vi "svx_SC Line Property Dialog.vi"(0 "Refnum":refnum<vi>, 1 "State In":T2={"X Scale"={"Name"="Horizontal", "format string"="%#.2g", "Major Color"=16777238, "Minor Color"=16777216, "Scale Visible"=TRUE, " Label Visible"=TRUE, "Grid Style"=1, "Maximum"=1.0, "Minimum"=-1.0}, "Y Scale"={"Name"="Vertical", "format string"="%#.2g", "Major Color"=16777238, "Minor Color"=16777216, "Scale Visible"=TRUE, " Label Visible"=TRUE, "Grid Style"=1, "Maximum"=1.0, "Minimum"=-1.0}, "Plot"={"Point Style"=0, "Line Width"=0, "Line Style"=0, "Plot Color"=16860, "Point/fill"=16860}, "Arrow Color"=16860, "Autoscale"=TRUE, "Property Name"=[], "Container Bounds"={"Width"=550, "Height"=313}, "Background color"=16777226, "Annotation List"=[], "Cursor"={"Cursor Point Style"=13, "Cursor Style"=4, "Cursor Line Width"=1, "Cursor Line Style"=0, "Cursor Color"=16711680, "Cursor Name Visible"=TRUE, "Cursor Visible"=TRUE, "Cursor Position"={"X"=0.0, "Y"=0.0}, "Cursor Index"=0, "Lock Cursor Name"=FALSE, "Cursor reference"=0.0}, "size"=0, "Boundary Color"=9868950, "Maximum"=1.0, "Marker Point Style"=2, "Maker Visible"=TRUE, "Marker Color"=16860, "pair strings []"=[], "clearance boundary"=[{"boundary"={"x axis"=0.0, "y axis"=0.0}, "start point"=enum."center"}], "Custom pair name"=FALSE, "selector.visible"=TRUE, "Cursor Release"=refnum, "Children Tags"=[], "open?"=TRUE, "pair index"=[], "Legend Width"=200, " Parents Tags"="", "Label"="", "Legend Background"=16777226, "Legend Font"=16777222, "scale fit"=2, "user strings []"=[], "Item Width"=0, "out of state queue"=refnum, "property nodes"=refnum, "Kind"=enum."X-Scale", "Scale Range Change"=refnum} caption="State" {"pair index" min=0; "Y Scale"."Minimum" min=0.0; "Y Scale"."Maximum" min=0.0; "X Scale"."Minimum" min=0.0; "X Scale"."Maximum" min=0.0}, 2 "Clearance Only?":bool, 5 "SC Line in":refnum<vi>, 7 "cursor info":refnum<vi>, 9 "Tree":refnum<vi>, 11 "Data":T1, 12 "Action in":T6 caption="Action") -> (3 "State Out":T2={"X Scale"={"Name"="Horizontal", "format string"="%#.2g", "Major Color"=16777238, "Minor Color"=16777216, "Scale Visible"=TRUE, " Label Visible"=TRUE, "Grid Style"=1, "Maximum"=1.0, "Minimum"=-1.0}, "Y Scale"={"Name"="Vertical", "format string"="%#.2g", "Major Color"=16777238, "Minor Color"=16777216, "Scale Visible"=TRUE, " Label Visible"=TRUE, "Grid Style"=1, "Maximum"=1.0, "Minimum"=-1.0}, "Plot"={"Point Style"=0, "Line Width"=0, "Line Style"=0, "Plot Color"=16860, "Point/fill"=16860}, "Arrow Color"=16860, "Autoscale"=TRUE, "Property Name"=[], "Container Bounds"={"Width"=550, "Height"=313}, "Background color"=16777226, "Annotation List"=[], "Cursor"={"Cursor Point Style"=13, "Cursor Style"=4, "Cursor Line Width"=1, "Cursor Line Style"=0, "Cursor Color"=16711680, "Cursor Name Visible"=TRUE, "Cursor Visible"=TRUE, "Cursor Position"={"X"=0.0, "Y"=0.0}, "Cursor Index"=0, "Lock Cursor Name"=FALSE, "Cursor reference"=0.0}, "size"=0, "Boundary Color"=9868950, "Maximum"=1.0, "Marker Point Style"=2, "Maker Visible"=TRUE, "Marker Color"=16860, "pair strings []"=[], "clearance boundary"=[{"boundary"={"x axis"=0.0, "y axis"=0.0}, "start point"=enum."center"}], "Custom pair name"=FALSE, "selector.visible"=TRUE, "Cursor Release"=refnum, "Children Tags"=[], "open?"=TRUE, "pair index"=[], "Legend Width"=200, " Parents Tags"="", "Label"="", "Legend Background"=16777226, "Legend Font"=16777222, "scale fit"=2, "user strings []"=[], "Item Width"=0, "out of state queue"=refnum, "property nodes"=refnum, "Kind"=enum."X-Scale", "Scale Range Change"=refnum} caption="State" {"pair index" min=0; "Y Scale"."Minimum" min=0.0; "Y Scale"."Maximum" min=0.0; "X Scale"."Minimum" min=0.0; "X Scale"."Maximum" min=0.0}, 14 "Action out":T6 caption="Action")   [LabVIEW 2017, in "SVX SC Line.xctl"]
uses:
  <vilib>/addons/_XControls/Shaft Centerline/SVX SC Line.xctl
  <vilib>/_xctls/Action.ctl
  <vilib>/addons/_XControls/Shaft Centerline/subVIs/svx_SC Line State.ctl
  <vilib>/addons/_XControls/Shaft Centerline/subVIs/svx_SC Line Bounds.ctl
  <vilib>/addons/_XControls/Shaft Centerline/subVIs/svx_SC Line Annotation List.ctl
  <vilib>/addons/_XControls/Shaft Centerline/subVIs/svx_SC Line OutState Queue.ctl
  <vilib>/addons/_XControls/Shaft Centerline/subVIs/svx_SC Line Data.ctl
  <vilib>/addons/_XControls/Shaft Centerline/subVIs/svx_SC Line Core States.ctl
  <vilib>/_xctls/XControlSupport.lvlib
panel:
  in  "Update Scale?":bool
  in  "Help":bool
  in  "Cancel":bool
  in  "OK":bool
  in  "Main Tab":T7(tab)
  in  "Legend Font.Color":u32(colorbox)=16777222 caption="Legend font"
  in  "Legend Background.Color":u32(colorbox)=16777226 caption="Legend background"
  in  "Background.Color":u32(colorbox)=16777226 caption="Background"
  in  "Direction.Color":u32(colorbox)=6618880 caption="Direction"
  in  "Label.Visible":bool=TRUE
  in  "Label.Text":string="Shaft Centerline"
  in  "Caption.Visible":bool
  in  "Caption.Text":string="Shaft Centerline"
  in  "Enable State":T8(radio)
  in  "Format Selection":u16(ring) items=["Horizontal (X-Axis)", "Vertical (Y-Axis)"]
  in  "Hide trailing zeros":bool=TRUE
  in  "Digits":u8=2
  in  "Precision Type":u16(ring) items=["Digits of precision", "Significant digits"]
  in  "Type":i32(listbox)=2
  in  "Plot.Point Style":T9={"OK Button 17"=TRUE, "OK Button"=FALSE, "OK Button 2"=FALSE, "OK Button 3"=FALSE, "OK Button 4"=FALSE, "OK Button 5"=FALSE, "OK Button 6"=FALSE, "OK Button 7"=FALSE, "OK Button 8"=FALSE, "OK Button 9"=FALSE, "OK Button 10"=FALSE, "OK Button 11"=FALSE, "OK Button 12"=FALSE, "OK Button 13"=FALSE, "OK Button 14"=FALSE, "OK Button 15"=FALSE, "OK Button 16"=FALSE} caption="Point Style"
  in  "Line.Color":u32(colorbox) caption="Line"
  in  "Plot.Line Style":T10={"OK Button"=TRUE, "OK Button 2"=FALSE, "OK Button 3"=FALSE, "OK Button 4"=FALSE, "OK Button 5"=FALSE} caption="Line Style"
  in  "Plot.Line Width":T11={"OK Button 2"=TRUE, "OK Button 3"=FALSE, "OK Button 4"=FALSE, "OK Button 5"=FALSE, "OK Button 6"=FALSE, "OK Button 7"=FALSE} caption="Line Width"
  in  "Point/Fill.Color":u32(colorbox)=16777226 caption="Point/Fill"
  in  "Marker.Point Style":T9 caption="Cursor Point Style"
  in  "Marker Color":u32(colorbox) caption="Marker"
  in  "Marker.Visible":bool=TRUE caption="Show marker"
  in  "YGrid Style":u16(ring) caption="Grid Style and Colors"
  in  "XGrid Style":u16(ring) caption="Grid Style and Colors"
  in  "Minor Grid.Color":u32(colorbox)=13056 caption="Minor grid"
  in  "Major Grid.Color":u32(colorbox)=26112 caption="Major grid"
  in  "Scale Label.Visible":bool caption="Show scale label"
  in  "Maximum":dbl=10.0 format="%0.2f"
  in  "Minimum":dbl format="%0.2f"
  in  "Scale Fit":bool caption="Autoscale"
  in  "Scale.Visible":bool=TRUE caption="Show scale"
  in  "Scale Name":string caption="Name"
  in  "Scale Selection":u16(ring) items=["Horizontal (X-Axis)", "Vertical (Y-Axis)"]
  in  "Cursor Info Position.Lock":bool=TRUE
  in  "Cursor.Line Width":T11 caption="Cursor Line Width"
  in  "Cursor.Point Style":T9 caption="Cursor Point Style"
  in  "Cursor.Line Style":T10 caption="Cursor Line Style"
  in  "Cursor Info.Visible":bool caption="Show name"
  in  "Cursor.Style":T12 caption="Cursor Style"
  in  "Cursor.Color":u32(colorbox) caption="Cursor color"
  in  "Cursor.Visible":bool=TRUE
  in  "Pair Selection":u16(ring)
  in  "Start Point":u16(ring)=2 caption="Start point" items=["Center", "Top", "Bottom"]
  in  "X Axis":dbl=0.02 caption="X axis" min=0.0
  in  "Y Axis":dbl=0.02 caption="Y axis" min=0.0
  in  "Clearance Boundary.Color":u32(colorbox)=14847 caption="Clearance boundary"
  in  "Tip strip":string
  in  "Description":string
  # "Caption"
  # "Label"
  # "Enabled State"
  # "Color Scheme"
  # "Shaft Centerline"
  # "Colors"
  # "Marker"
  # "Cursor"
  # "Boundary"
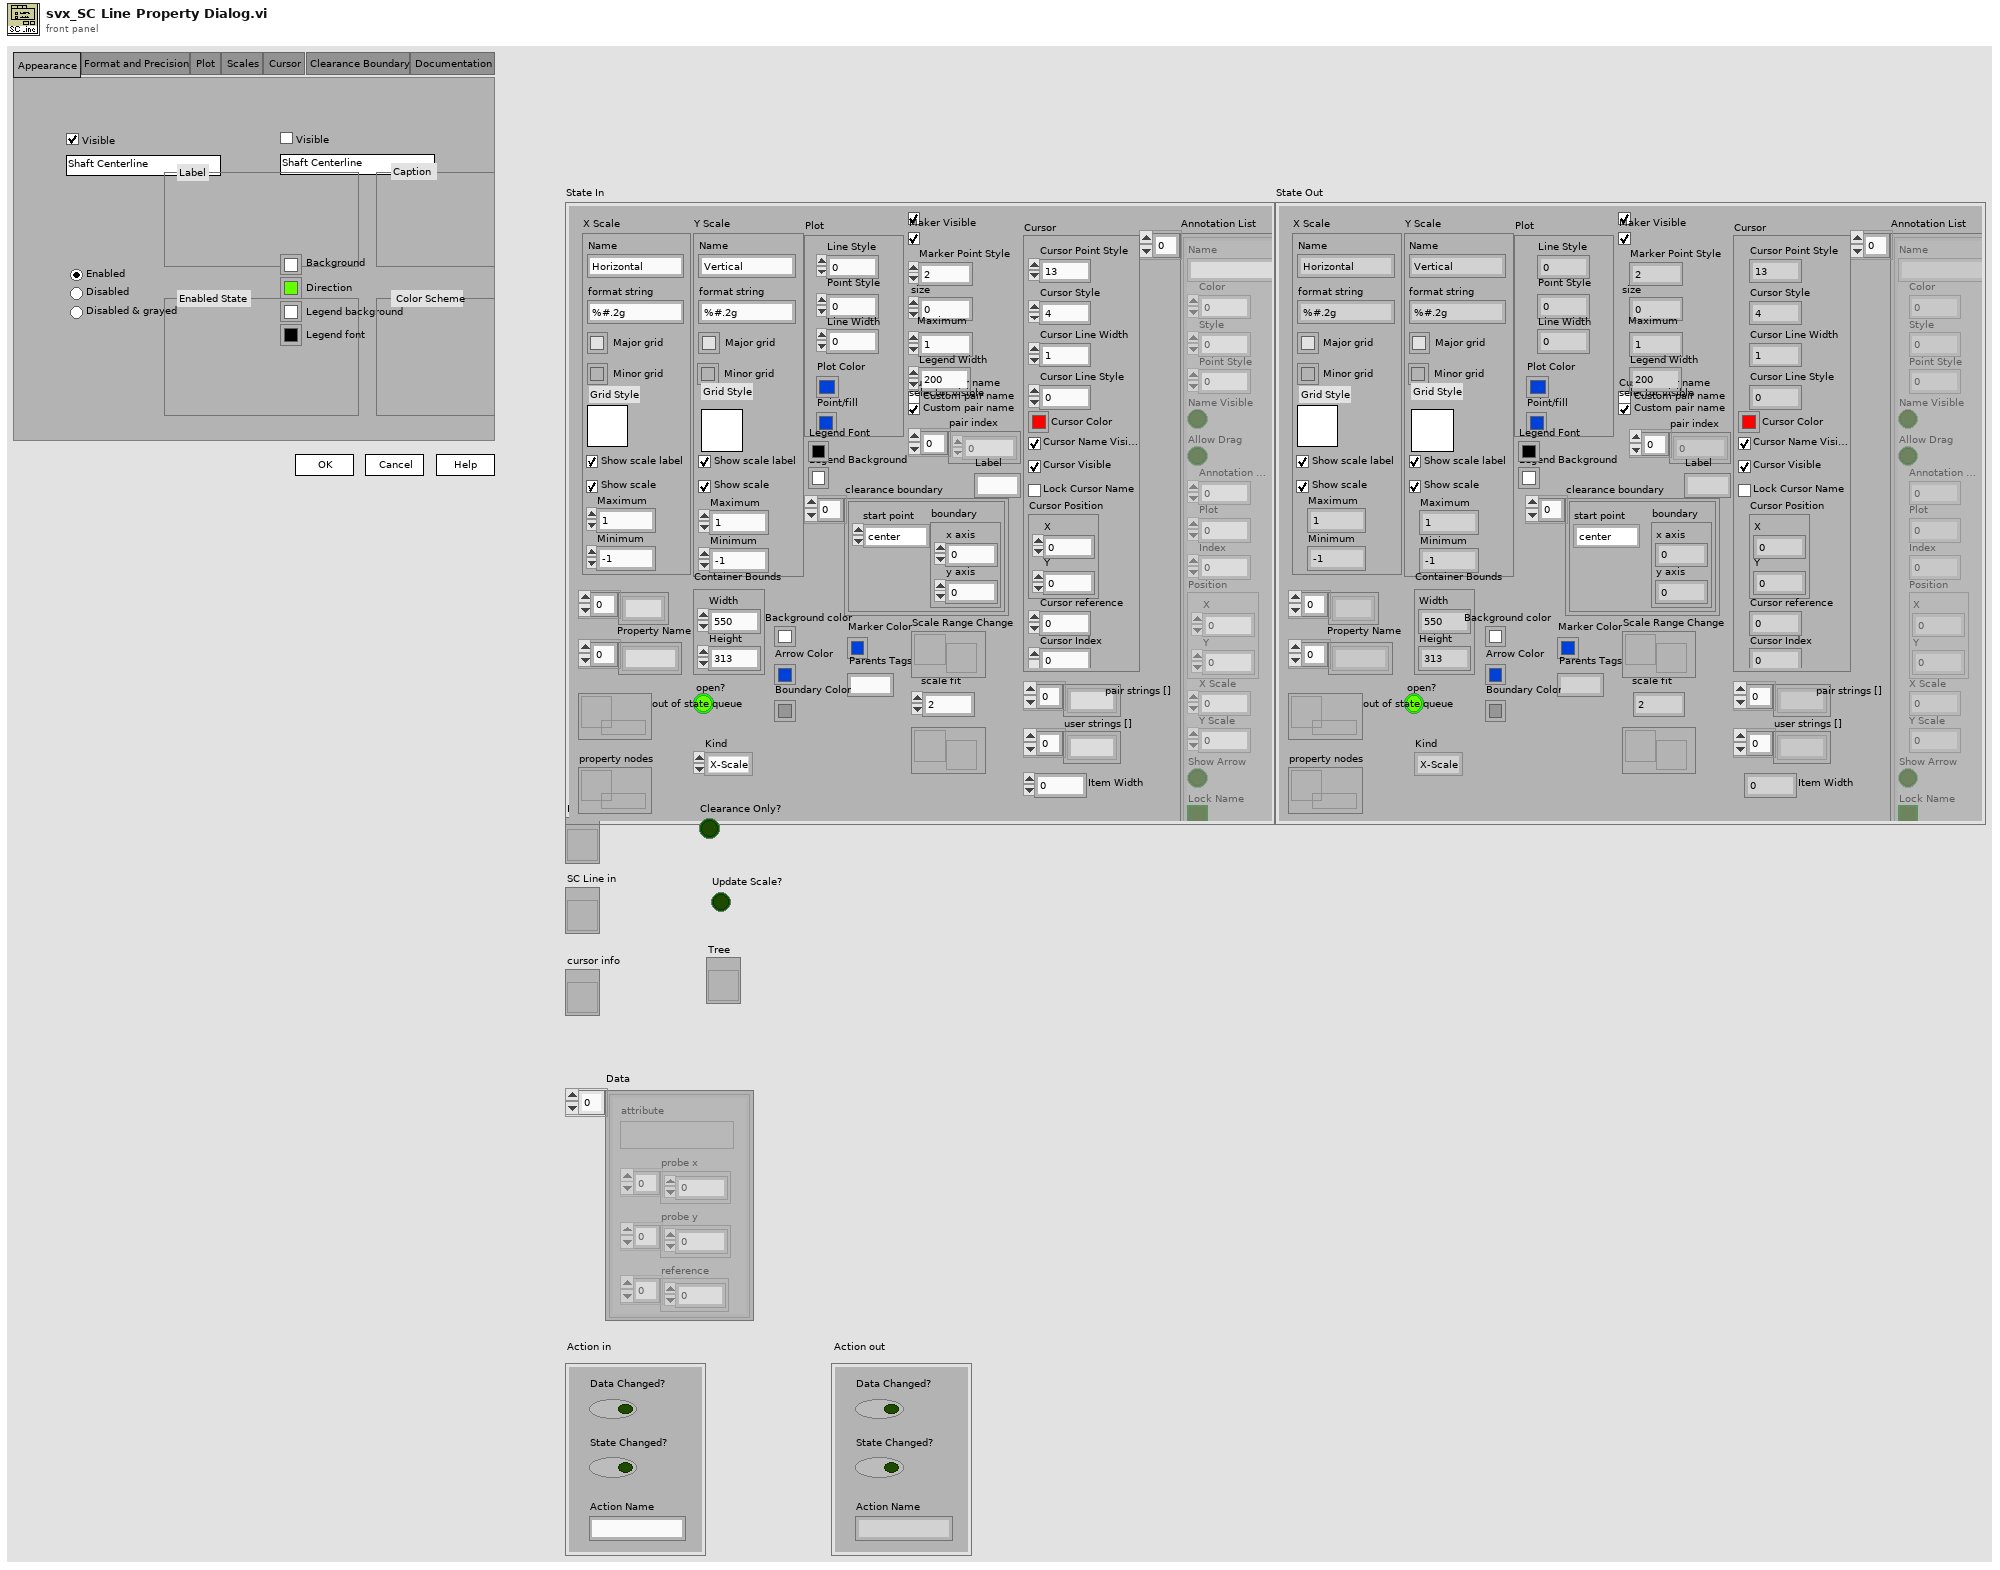
[diagram p1: front panel]
types:
  T1 = typedef "SVX SC Line.xctl/svx_SC Line Data.ctl" = cluster{"probe x":dbl[], "probe y":dbl[], "reference":dbl[], "attribute":variant}[]
  T2 = typedef "SVX SC Line.xctl/svx_SC Line State.ctl" = cluster{"X Scale":cluster{"Name":string, "format string":string, "Major Color":u32, "Minor Color":u32, "Scale Visible":bool, " Label Visible":bool, "Grid Style":u16, "Maximum":dbl, "Minimum":dbl}, "Y Scale":cluster{"Name":string, "format string":string, "Major Color":u32, "Minor Color":u32, "Scale Visible":bool, " Label Visible":bool, "Grid Style":u16, "Maximum":dbl, "Minimum":dbl}, "Plot":cluster{"Point Style":u8, "Line Width":u8, "Line Style":u8, "Plot Color":u32, "Point/fill":u32}, "Arrow Color":u32, "Autoscale":bool, "Property Name":string[], "Container Bounds":T3, "Background color":u32, "Annotation List":T4, "Cursor":cluster{"Cursor Point Style":u8, "Cursor Style":u8, "Cursor Line Width":u8, "Cursor Line Style":u8, "Cursor Color":u32, "Cursor Name Visible":bool, "Cursor Visible":bool, "Cursor Position":cluster{"X":dbl, "Y":dbl}, "Cursor Index":i32, "Lock Cursor Name":bool, "Cursor reference":dbl}, "size":i32, "Boundary Color":u32, "Maximum":dbl, "Marker Point Style":u8, "Maker Visible":bool, "Marker Color":u32, "pair strings []":string[], "clearance boundary":cluster{"boundary":cluster{"x axis":dbl, "y axis":dbl}, "start point":enum16{"center", "top", "bottom"}}[], "Custom pair name":bool, "selector.visible":bool, "Cursor Release":refnum<user-event>, "Children Tags":string[], "open?":bool, "pair index":i32[], "Legend Width":u32, " Parents Tags":string, "Label":string, "Legend Background":u32, "Legend Font":u32, "scale fit":u8, "user strings []":string[], "Item Width":u32, "out of state queue":T5, "property nodes":refnum<queue>, "Kind":enum16{"X-Scale", "Y-Scale", "Z-Scale"}, "Scale Range Change":refnum<user-event>}
  T3 = typedef "SVX SC Line.xctl/svx_SC Line Bounds.ctl" = cluster{"Width":u32, "Height":u32}
  T4 = typedef "SVX SC Line.xctl/svx_SC Line Annotation List.ctl" = cluster{"Name":string, "Color":u32, "Style":u8, "Point Style":u8, "Name Visible":bool, "Allow Drag":bool, "Annotation Mode":u32, "Plot":i32, "Index":i32, "Position":cluster{"X":dbl, "Y":dbl}, "X Scale":u32, "Y Scale":u32, "Show Arrow":bool, "Lock Name":bool, "Plot Area":i32, "Label Offset":cluster{"X":dbl, "Y":dbl}}[]
  T5 = typedef "SVX SC Line.xctl/svx_SC Line OutState Queue.ctl" = refnum<queue>
  T6 = typedef "XControlSupport.lvlib/Action.ctl" = cluster{"Data Changed?":bool, "State Changed?":bool, "Action Name":string}
  T7 = enum32{"Appearance", "Format and Precision", "Plot", "Scales", "Cursor", "Clearance Boundary", "Documentation"}
  T8 = enum32{"Enabled", "Disabled", "Disabled & grayed"}
  T9 = cluster{"OK Button 17":bool, "OK Button":bool, "OK Button 2":bool, "OK Button 3":bool, "OK Button 4":bool, "OK Button 5":bool, "OK Button 6":bool, "OK Button 7":bool, "OK Button 8":bool, "OK Button 9":bool, "OK Button 10":bool, "OK Button 11":bool, "OK Button 12":bool, "OK Button 13":bool, "OK Button 14":bool, "OK Button 15":bool, "OK Button 16":bool}
  T10 = cluster{"OK Button":bool, "OK Button 2":bool, "OK Button 3":bool, "OK Button 4":bool, "OK Button 5":bool}
  T11 = cluster{"OK Button 2":bool, "OK Button 3":bool, "OK Button 4":bool, "OK Button 5":bool, "OK Button 6":bool, "OK Button 7":bool}
  T12 = cluster{"OK Button 17":bool, "OK Button":bool, "OK Button 2":bool, "OK Button 5":bool, "OK Button 13":bool, "OK Button 10":bool, "OK Button 6":bool, "OK Button 9":bool, "OK Button 14":bool}
  T13 = cluster{"boundary":cluster{"x axis":dbl, "y axis":dbl}, "start point":enum16{"center", "top", "bottom"}}[]
  T14 = cluster{"boundary":cluster{"x axis":dbl, "y axis":dbl}, "start point":enum16{"center", "top", "bottom"}}
  T15 = cluster{"Desc":string, "TipStrip":string, "Label.Text":string, "Label.Visible":bool, "Caption.Text":string, "Caption.Visible":bool, "Disabled":u8}
  T16 = cluster{"Refnum":refnum<vi>, "SC Line in":refnum<vi>, "cursor info":refnum<vi>, "Tree":refnum<vi>, "This VI":refnum<vi>}
  T17 = typedef "SVX SC Line.xctl/svx_SC Line Core States.ctl" = enum16{"None", "[Axis] Autoscale", "[Image] Update", "[Cursor] Name", "[Plot] Grid&BG", "[Marker] Update", "[Tree] Tags", "[Data] Update", "[Layout] Size", "[Tree] Checkbox", "[Tree] Visible", "[Tree] Open", "[Axis] X", "[Axis] Y", "[Plot] Color", "[Axis] Format String", "[Data] Compare Strings", "[Cursor] Apearance", "[Axis] Name&Visible", "[Tree] Color", "[Data] Index", "[Cursor] Index", "[Axis] Event"}
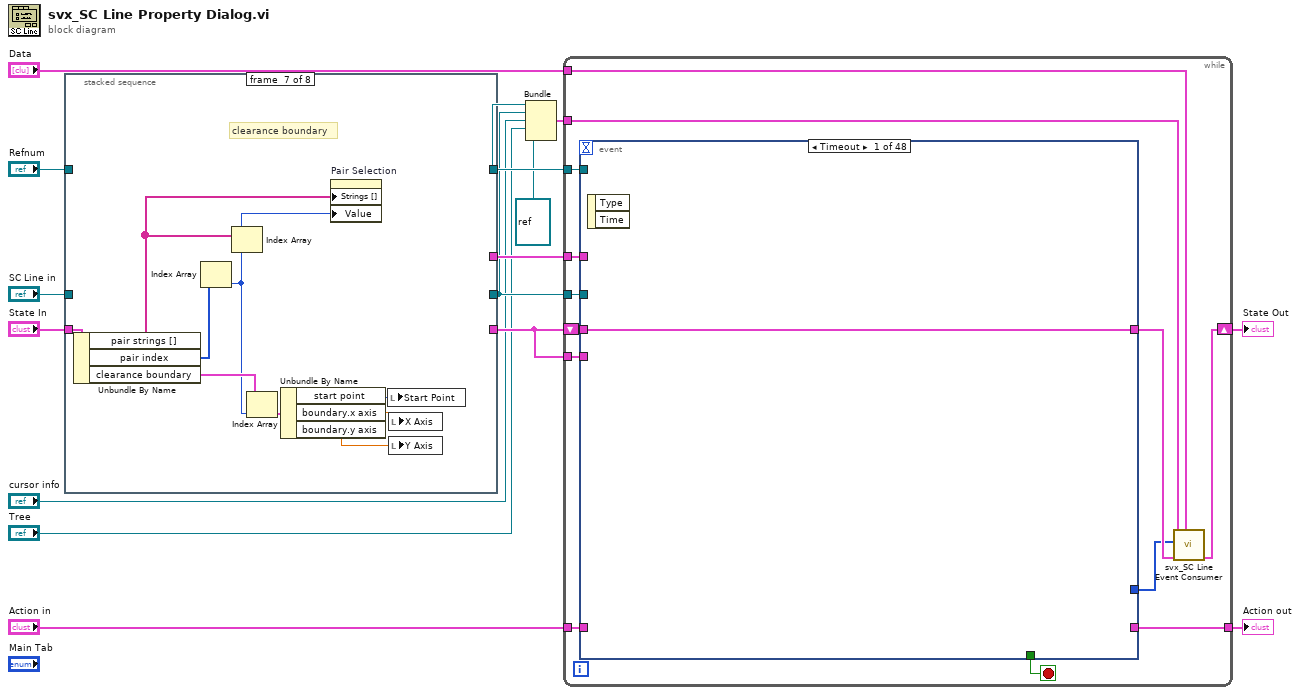
[diagram p0: block diagram]
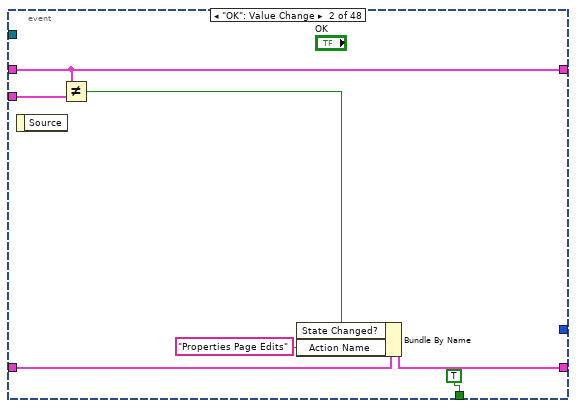
[diagram p2: hidden frame]
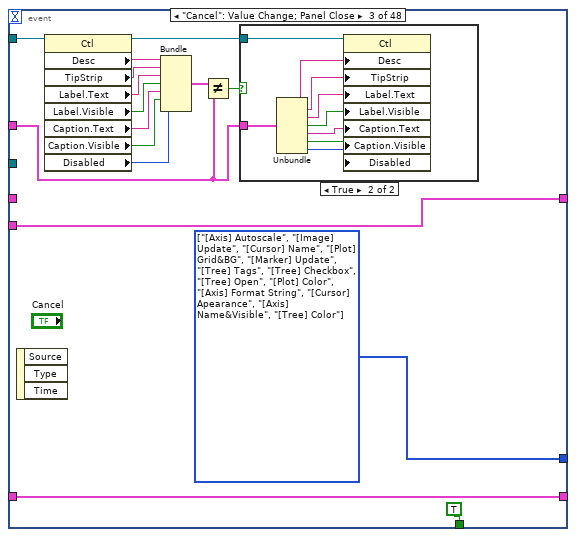
[diagram p3: hidden frame]
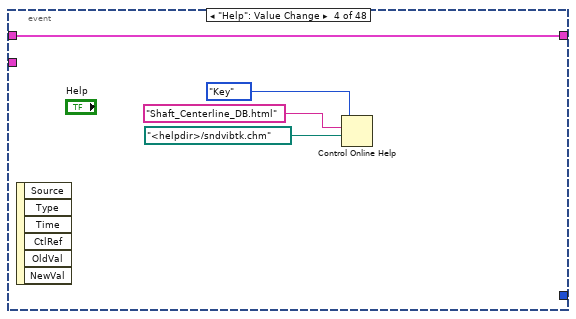
[diagram p5: hidden frame]
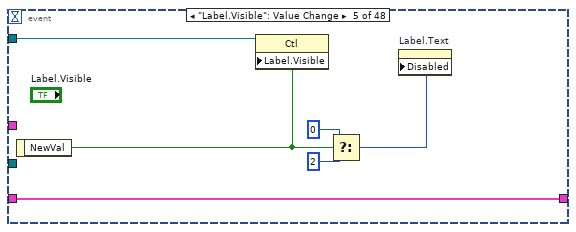
[diagram p6: hidden frame]
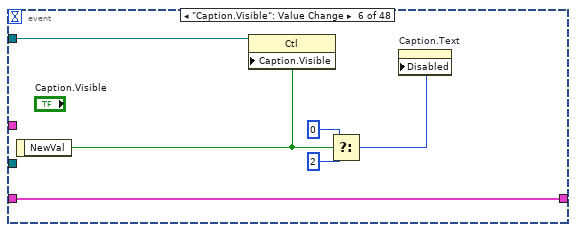
[diagram p7: hidden frame]
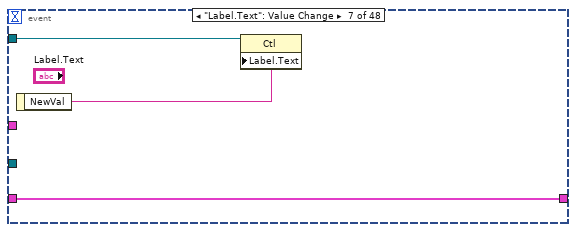
[diagram p8: hidden frame]
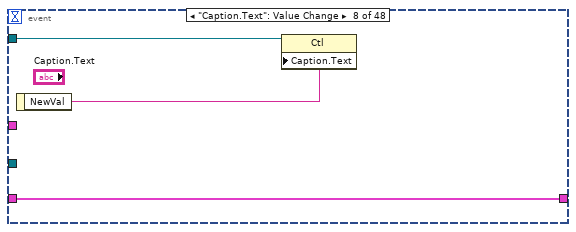
[diagram p9: hidden frame]
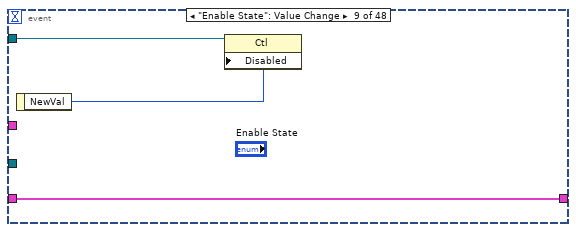
[diagram p10: hidden frame]
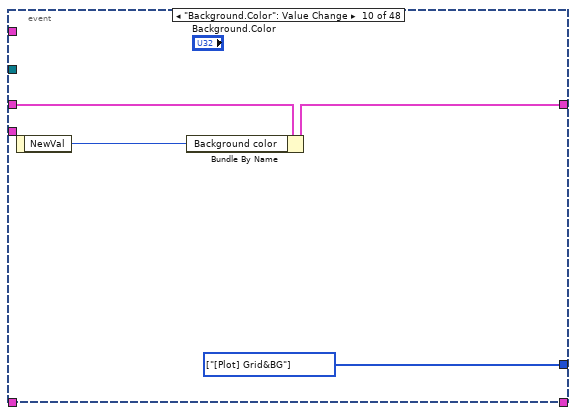
[diagram p11: hidden frame]
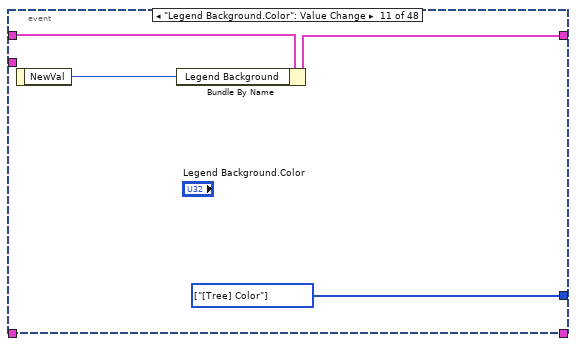
[diagram p12: hidden frame]
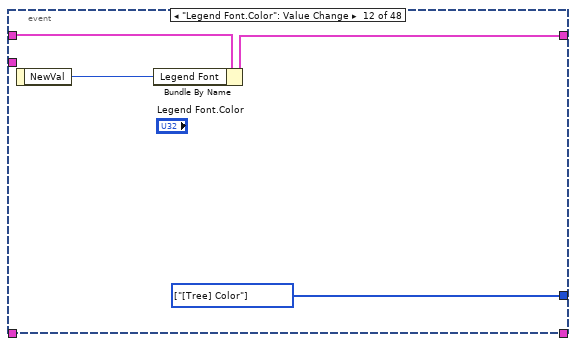
[diagram p13: hidden frame]
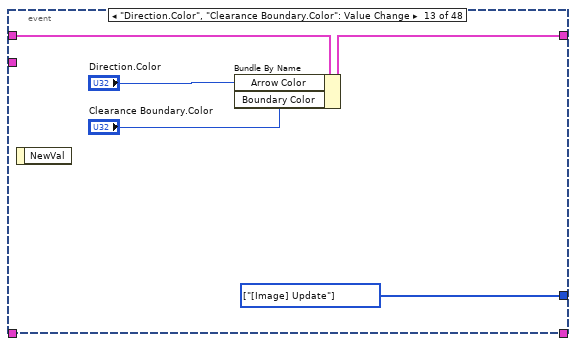
[diagram p14: hidden frame]
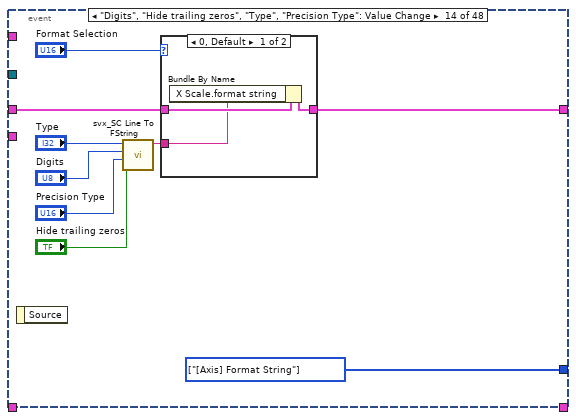
[diagram p15: hidden frame]
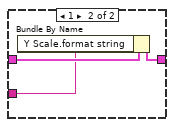
[diagram p16: hidden frame]
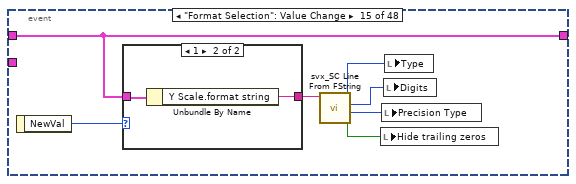
[diagram p17: hidden frame]
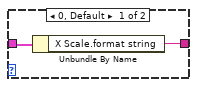
[diagram p18: hidden frame]
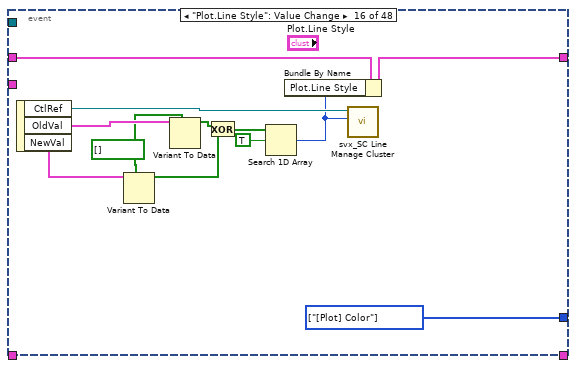
[diagram p19: hidden frame]
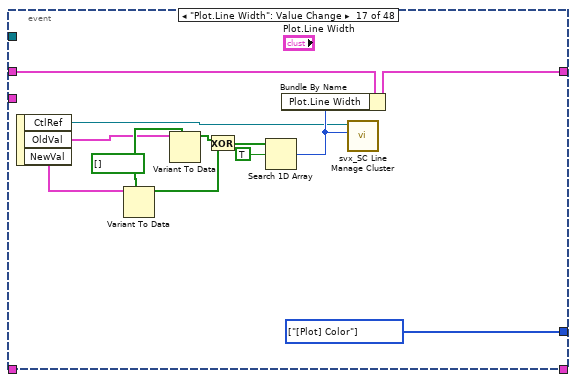
[diagram p20: hidden frame]
diagram:
  n1 = stacked-sequence {
    tunnel: "Refnum" -> [_ w47 _ _ _ _ _ w144]
    tunnel: [_ _ _ _ _ _ _ w143] -> w6
    tunnel: [_ _ _ _ _ _ _ w140] -> w14
    tunnel: [_ _ _ _ _ _ _ w141] -> w5
    tunnel: "SC Line in" -> [_ _ _ _ _ _ _ w141]
    tunnel: [_ _ _ _ _ _ _ w142] -> w11
    tunnel: "State In" -> [_ w30 w48 w58 w67 w100 w124 w140]
    frame #0 {
      n2 = property on="Main Tab" class="TabCtl (strict)"() -> ("Pages"=w18:refnum<vi>[])  [unwired: 2 in, 2 out]
      n3 = case shown="True" "Clearance Only?" {
        tunnel: w18 -> [w21 w27]
        tunnel: [T7."Clearance Boundary" ("Main Tab") T7."Appearance" ("Main Tab")] -> w17
        frame True {
          n4 = for {
            tunnel: w21 -> [w25] mode=indexing
            i -> [w24]
            n5 = Equal?(x=5, y=w24) -> (x = y?=w22:bool)
            n6 = property on="Property Node" class="Page"(reference=w25, "PageVis"=w22) -> ()  [unwired: 1 in, 2 out]
          }
        }
        frame False {
          n7 = for {
            tunnel: w27 -> [w29] mode=indexing
            n8 = property on="Property Node" class="Page"(reference=w29, "PageVis"=TRUE ("Page Visible")) -> ()  [unwired: 1 in, 2 out]
          }
        }
      }
      n9 = local write "Main Tab"(w17) -> ()
      n10 = local write "Update Scale?"(FALSE ("Update Scale?")) -> ()
    }
    frame #1 {
      # "Appearance"
      n11 = Unbundle By Name(w30) -> ("Background color"=w46:u32, "Arrow Color"=w45:u32, "Boundary Color"=w33:u32, "Legend Background"=w32:u32, "Legend Font"=w31:u32)
      n12 = property class="Ctl"(reference=w47) -> ("Label.Text"=w39:string, "Label.Visible"=w38:bool, "Caption.Text"=w37:string, "Caption.Visible"=w35:bool, "Disabled"=w36:u8)  [unwired: 1 in, 2 out]
      n13 = local write "Clearance Boundary.Color"(w33) -> ()
      n14 = local write "Background.Color"(w46) -> ()
      n15 = local write "Legend Font.Color"(w31) -> ()
      n16 = local write "Caption.Text"(w37) -> ()
      n17 = local write "Label.Text"(w39) -> ()
      n18 = local write "Enable State"(w36) -> ()
      n19 = local write "Caption.Visible"(w35) -> ()
      n20 = local write "Label.Visible"(w38) -> ()
      n21 = local write "Legend Background.Color"(w32) -> ()
      n22 = local write "Direction.Color"(w45) -> ()
      n23 = Select(t=u8 0 ("Disabled"), s=w38, f=u8 2) -> (s? t:f=w43:u8)
      n24 = Select(t=u8 0 ("Disabled"), s=w35, f=u8 2) -> (s? t:f=w40:u8)
      n25 = property on="Label.Text" class="Str"("Disabled"=w43) -> ()  [unwired: 2 in, 2 out]
      n26 = property on="Caption.Text" class="Str"("Disabled"=w40) -> ()  [unwired: 2 in, 2 out]
    }
    frame #2 {
      w54 = u16 0 items=["X-Axis", "Y-Axis"] ("Format selection")
      # "Format and Precision"
      n27 = Unbundle By Name(w48) -> ("X Scale.format string"=w53:string)
      n28 = call <vilib>:"svx_SC Line From FString.vi"("Format string"=w53) -> ("trailing zeros"=w49:bool, "Precision Type"=w50:u16, "Digits"=w51:u8, "Type"=w52:i32)  [unwired: 7 in]
      n29 = local write "Format Selection"(w54) -> ()
      n30 = local write "Hide trailing zeros"(w49) -> ()
      n31 = local write "Precision Type"(w50) -> ()
      n32 = local write "Digits"(w51) -> ()
      n33 = local write "Type"(w52) -> ()
    }
    frame #3 {
      # "Plot"
      n34 = Unbundle By Name(w58) -> ("Plot.Plot Color"=w60:u32, "Plot.Point/fill"=w59:u32, "Plot.Line Width"=w66:u8, "Plot.Line Style"=w64:u8, "Plot.Point Style"=w63:u8)
      n35 = control-ref of="Plot.Line Width"() -> (w65:refnum<vi>)
      n36 = control-ref of="Plot.Line Style"() -> (w61:refnum<vi>)
      n37 = control-ref of="Plot.Point Style"() -> (w62:refnum<vi>)
      n38 = local write "Line.Color"(w60) -> ()
      n39 = To Long Integer(number=w66) -> (32bit integer=w55:i32)
      n40 = To Long Integer(number=w64) -> (32bit integer=w56:i32)
      n41 = To Long Integer(number=w63) -> (32bit integer=w57:i32)
      n42 = local write "Point/Fill.Color"(w59) -> ()
      n43 = call <vilib>:"svx_SC Line Manage Cluster.vi"("index"=w55, "Clust Refnum"=w65) -> ()  [unwired: 10 in]
      n44 = call <vilib>:"svx_SC Line Manage Cluster.vi"("index"=w56, "Clust Refnum"=w61) -> ()  [unwired: 10 in]
      n45 = call <vilib>:"svx_SC Line Manage Cluster.vi"("index"=w57, "Clust Refnum"=w62) -> ()  [unwired: 10 in]
    }
    frame #4 {
      w90 = u16 0 items=["X-Axis", "Y-Axis"] ("Scale selection")
      # "Scales"
      n46 = Unbundle By Name(w67) -> ("Y Scale.Name"=w73:string, "X Scale.Name"=w71:string, "X Scale.Label Visible"=w89:bool, "X Scale.Scale Visible"=w88:bool, "X Scale.Grid Style"=w78:u16, "X Scale.Major Color"=w87:u32, "X Scale.Minor Color"=w86:u32, "Autoscale"=w83:bool, "X Scale.Minimum"=w76:dbl, "X Scale.Maximum"=w75:dbl)
      n47 = property on="YGrid Style" class="Ring (strict)"("Visible"=FALSE) -> ()  [unwired: 2 in, 2 out]
      n48 = property on="XGrid Style" class="Ring (strict)"("Visible"=TRUE) -> ()  [unwired: 2 in, 2 out]
      n49 = Concatenate Strings(w73, " (Y-Axis)" ("string")) -> (w69:string)
      n50 = Concatenate Strings(w71, " (X-Axis)" ("string")) -> (w70:string)
      n51 = local write "Minimum"(w76) -> ()
      n52 = local write "Scale Label.Visible"(w89) -> ()
      n53 = local write "Maximum"(w75) -> ()
      n54 = local write "Minor Grid.Color"(w86) -> ()
      n55 = local write "XGrid Style"(w78) -> ()
      n56 = local write "Scale Selection"(w90) -> ()
      n57 = case shown="0, Default" w78 {
        tunnel: [w91 u8 0 ("Disabled") w94] -> w80
        tunnel: [w91 u8 2 ("Disabled") w94] -> w79
        frame 0, Default {
          w91 = u8 2 ("Disabled")
        }
        frame 1 {
        }
        frame 2 {
          w94 = u8 0 ("Disabled")
        }
      }
      n58 = Build Array(w70, w69) -> (w68:string[])
      n59 = property on="Scale Selection" class="Ring (strict)"("Strings []"=w68) -> ()  [unwired: 2 in, 2 out]
      n60 = property on="Format Selection" class="Ring (strict)"("Strings []"=w68) -> ()  [unwired: 2 in, 2 out]
      n61 = Select(t=u8 2 ("Disabled"), s=w83, f=u8 0) -> (s? t:f=w82:u8)
      n62 = local write "Scale Name"(w71) -> ()
      n63 = local write "Scale.Visible"(w88) -> ()
      n64 = local write "Major Grid.Color"(w87) -> ()
      n65 = local write "Scale Fit"(w83) -> ()
      n66 = property on="Minimum" class="DigNum (strict)"("Disabled"=w82) -> ()  [unwired: 2 in, 2 out]
      n67 = property on="Maximum" class="DigNum (strict)"("Disabled"=w82) -> ()  [unwired: 2 in, 2 out]
      n68 = property on="Major Grid.Color" class="ColBox"("Disabled"=w80) -> ()  [unwired: 2 in, 2 out]
      n69 = property on="Minor Grid.Color" class="ColBox"("Disabled"=w79) -> ()  [unwired: 2 in, 2 out]
    }
    frame #5 {
      # "Cursor"
      n70 = Unbundle By Name(w100) -> ("Cursor.Cursor Point Style"=w123:u8, "Cursor.Cursor Style"=w121:u8, "Cursor.Cursor Line Width"=w119:u8, "Cursor.Cursor Line Style"=w117:u8, "Cursor.Cursor Color"=w115:u32, "Cursor.Cursor Name Visible"=w102:bool, "Cursor.Cursor Visible"=w103:bool, "Marker Point Style"=w114:u8, "Maker Visible"=w112:bool, "Marker Color"=w111:u32, "Cursor.Lock Cursor Name"=w110:bool)
      n71 = And(x=w103, y=w102) -> (x .and. y?=w101:bool)
      n72 = Select(t=u8 0 ("Disabled"), s=w101, f=u8 2) -> (s? t:f=w104:u8)
      n73 = Select(t=u8 0 ("Disabled"), s=w103, f=u8 2) -> (s? t:f=w107:u8)
      n74 = property on="Cursor Info.Visible" class="Bool (strict)"("Disabled"=w107) -> ()  [unwired: 2 in, 2 out]
      n75 = property on="Cursor Info Position.Lock" class="Bool (strict)"("Disabled"=w104) -> ()  [unwired: 2 in, 2 out]
      n76 = local write "Cursor Info Position.Lock"(w110) -> ()
      n77 = local write "Cursor.Visible"(w103) -> ()
      n78 = local write "Marker.Visible"(w112) -> ()
      n79 = local write "Cursor.Color"(w115) -> ()
      n80 = To Long Integer(number=w121) -> (32bit integer=w96:i32)
      n81 = To Long Integer(number=w117) -> (32bit integer=w98:i32)
      n82 = control-ref of="Cursor.Point Style"() -> (w122:refnum<vi>)
      n83 = control-ref of="Cursor.Style"() -> (w120:refnum<vi>)
      n84 = control-ref of="Cursor.Line Style"() -> (w116:refnum<vi>)
      n85 = call <vilib>:"svx_SC Line Manage Cluster.vi"("index"=w96, "Clust Refnum"=w120) -> ()  [unwired: 10 in]
      n86 = call <vilib>:"svx_SC Line Manage Cluster.vi"("index"=w98, "Clust Refnum"=w116) -> ()  [unwired: 10 in]
      n87 = To Long Integer(number=w119) -> (32bit integer=w97:i32)
      n88 = To Long Integer(number=w114) -> (32bit integer=w99:i32)
      n89 = local write "Cursor Info.Visible"(w102) -> ()
      n90 = To Long Integer(number=w123) -> (32bit integer=w95:i32)
      n91 = control-ref of="Marker.Point Style"() -> (w113:refnum<vi>)
      n92 = local write "Marker Color"(w111) -> ()
      n93 = control-ref of="Cursor.Line Width"() -> (w118:refnum<vi>)
      n94 = call <vilib>:"svx_SC Line Manage Cluster.vi"("index"=w99, "Clust Refnum"=w113) -> ()  [unwired: 10 in]
      n95 = call <vilib>:"svx_SC Line Manage Cluster.vi"("index"=w95, "Clust Refnum"=w122) -> ()  [unwired: 10 in]
      n96 = call <vilib>:"svx_SC Line Manage Cluster.vi"("index"=w97, "Clust Refnum"=w118) -> ()  [unwired: 10 in]
    }
    frame #6 {
      # "clearance boundary"
      n97 = Unbundle By Name(w124) -> ("pair strings []"=w125:string[], "pair index"=w127:i32[], "clearance boundary"=w132:T13)
      n98 = Index Array(array=w127) -> (element=w126:i32)  [unwired: 1 in]
      n99 = Index Array(array=w125, index=w126) -> ()  [unwired: 1 out]
      n100 = Index Array(array=w132, index=w126) -> (element=w131:T14)
      n101 = Unbundle By Name(w131) -> ("start point"=w130:enum16{"center", "top", "bottom"}, "boundary.x axis"=w128:dbl, "boundary.y axis"=w129:dbl)
      n102 = property on="Pair Selection" class="Ring (strict)"("Strings []"=w125, "Value"=w126) -> ()  [unwired: 2 in, 2 out]
      n103 = local write "Start Point"(w130) -> ()
      n104 = local write "X Axis"(w128) -> ()
      n105 = local write "Y Axis"(w129) -> ()
    }
    frame #7 {
      n106 = property class="Ctl"(reference=w144) -> (reference out=w143:refnum<vi>, "Desc"=w133:string, "TipStrip"=w134:string, "Label.Text"=w139:string, "Label.Visible"=w138:bool, "Caption.Text"=w137:string, "Caption.Visible"=w136:bool, "Disabled"=w135:u8)  [unwired: 1 in, 1 out]
      n107 = local write "Description"(w133) -> ()
      n108 = local write "Tip strip"(w134) -> ()
      n109 = Bundle("Desc"=w133, "TipStrip"=w134, "Label.Text"=w139, "Label.Visible"=w138, "Caption.Text"=w137, "Caption.Visible"=w136, "Disabled"=w135) -> (w142:T15)  [unwired: 1 in]
    }
  }
  n110 = Bundle("Refnum"=w6, "SC Line in"=w5, "cursor info"="cursor info", "Tree"="Tree", "This VI"=refnum<vi> refnum) -> (w4:T16)  [unwired: 1 in]
  n111 = while {
    tunnel: w6 -> [w147]
    shift-right: [w150] -> w10
    shift-left: w14 -> [w156]
    tunnel: w14 -> [w153]
    tunnel: "Action in" -> [w152]
    tunnel: [w155] -> w12
    tunnel: w5 -> [w146]
    tunnel: w11 -> [w154]
    tunnel: "Data" -> [w148]
    tunnel: w4 -> [w145]
    stop <- w157 stop-if-true
    n112 = event shown="[0] Timeout" {
      selector: _ -> [_ _ _ _ _ _ _ _ _ _ _ _ _ _ _ _ _ _ _ _ _ _ _ _ _ _ _ _ _ _ _ _ _ _ _ _ _ _ _ _ _ _ _ _ _ _ _ _]
      dyn-events: _ -> [_ _ _ _ _ _ _ _ _ _ _ _ _ _ _ _ _ _ _ _ _ _ _ _ _ _ _ _ _ _ _ _ _ _ _ _ _ _ _ _ _ _ _ _ _ _ _ _]
      timeout: _ -> [_ _ _ _ _ _ _ _ _ _ _ _ _ _ _ _ _ _ _ _ _ _ _ _ _ _ _ _ _ _ _ _ _ _ _ _ _ _ _ _ _ _ _ _ _ _ _ _]
      tunnel: [_ TRUE TRUE _ _ _ _ _ _ _ _ _ _ _ _ _ _ _ _ _ _ _ _ _ _ _ _ _ _ _ _ _ _ _ _ _ _ _ _ _ _ _ _ _ _ _ _ _] -> w157
      tunnel: w156 -> [w158 w159 _ w191 w195 w201 w207 w210 w213 w219 w223 w227 w229 w235 w253 w262 w277 w289 w298 w302 w311 w324 w335 w351 w366 w386 w396 w406 w417 w427 w474 w486 w498 w510 w522 w526 w538 w542 w549 w558 w562 w573 w588 w603 w608 w615 w618 w621]
      tunnel: w153 -> [_ w164 w179 _ _ _ _ _ _ _ _ _ _ _ _ _ _ _ _ _ _ _ _ _ _ _ _ _ _ _ _ _ _ _ _ _ _ _ _ _ _ _ _ _ _ _ _ _]
      tunnel: [_ w162 w181 _ _ _ _ _ _ _ _ _ _ _ _ _ _ _ _ _ _ _ _ _ _ _ _ _ _ _ _ _ _ _ _ _ _ _ _ _ _ _ _ _ _ _ _ _] -> w155
      tunnel: [_ _ w166 _ _ _ _ _ _ w216 w220 w224 w228 w233 _ w259 w271 w283 w295 w299 w303 w320 w331 w348 w364 w382 w392 w402 w413 _ w468 w480 w492 w504 w516 w523 w527 w539 w543 w555 w559 w568 w583 w598 _ _ _ _] -> w149
      tunnel: w146 -> [_ _ _ _ _ _ _ _ _ _ _ _ _ _ _ _ _ _ _ _ _ _ _ w349 _ _ _ _ _ _ _ _ _ _ _ _ _ _ _ _ _ _ _ _ _ _ _ _]
      tunnel: w147 -> [_ _ w178 _ w200 w206 w209 w212 w215 _ _ _ _ _ _ _ _ _ _ _ _ _ _ _ _ _ _ _ _ _ _ _ _ _ _ _ _ _ _ _ _ _ _ _ _ w617 w620 _]
      tunnel: w154 -> [_ _ w169 _ _ _ _ _ _ _ _ _ _ _ _ _ _ _ _ _ _ _ _ _ _ _ _ _ _ _ _ _ _ _ _ _ _ _ _ _ _ _ _ _ _ _ _ _]
      tunnel: [w158 w159 w179 w191 w195 w201 w207 w210 w213 w218 w222 w226 w232 w234 w253 w261 w276 w288 w297 w301 w310 w323 w334 w347 w365 w387 w397 w405 w416 w427 w473 w485 w497 w509 w521 w525 w537 w541 w548 w557 w561 w572 w587 w602 w608 w615 w618 w621] -> w151
      tunnel: w152 -> [_ w163 w181 _ _ _ _ _ _ _ _ _ _ _ _ _ _ _ _ _ _ _ _ _ _ _ _ _ _ _ _ _ _ _ _ _ _ _ _ _ _ _ _ _ _ _ _ _]
      event Timeout {
        n113 = event-data() -> ()  [unwired: 1 in, 2 out]
      }
      event "OK": Value Change {
        n114 = event-data() -> ()  [unwired: 1 in, 1 out]
        n115 = Not Equal?(x=w159, y=w164) -> (x != y?=w161:bool)
        n116 = Bundle By Name(cluster=w163, "State Changed?"=w161, "Action Name"="Properties Page Edits") -> (w162:T6)
      }
      event "Cancel": Value Change; Panel Close {
        w166 = T17[] [enum."[Axis] Autoscale", enum."[Image] Update", enum."[Cursor] Name", enum."[Plot] Grid&BG", enum."[Marker] Update", enum."[Tree] Tags", enum."[Tree] Checkbox", enum."[Tree] Open", enum."[Plot] Color", enum."[Axis] Format String", enum."[Cursor] Apearance", enum."[Axis] Name&Visible", enum."[Tree] Color"] items=["None", "[Axis] Autoscale", "[Image] Update", "[Cursor] Name", "[Plot] Grid&BG", "[Marker] Update", "[Tree] Tags", "[Data] Update", "[Layout] Size", "[Tree] Checkbox", "[Tree] Visible", "[Tree] Open", "[Axis] X", "[Axis] Y", "[Plot] Color", "[Axis] Format String", "[Data] Compare Strings", "[Cursor] Apearance", "[Axis] Name&Visible", "[Tree] Color", "[Data] Index", "[Cursor] Index", "[Axis] Event"]
        n117 = event-data() -> ()  [unwired: 1 in, 3 out]
        n118 = property class="Ctl"(reference=w178) -> (reference out=w168:refnum<vi>, "Desc"=w177:string, "TipStrip"=w176:string, "Label.Text"=w175:string, "Label.Visible"=w174:bool, "Caption.Text"=w173:string, "Caption.Visible"=w172:bool, "Disabled"=w171:u8)  [unwired: 1 in, 1 out]
        n119 = Bundle("Desc"=w177, "TipStrip"=w176, "Label.Text"=w175, "Label.Visible"=w174, "Caption.Text"=w173, "Caption.Visible"=w172, "Disabled"=w171) -> (w170:T15)  [unwired: 1 in]
        n120 = Not Equal?(x=w170, y=w169) -> (x != y?=w167:bool)
        n121 = case shown="True" w167 {
          tunnel: w169 -> [_ w190]
          tunnel: w168 -> [_ w182]
          frame False {
          }
          frame True {
            n122 = Unbundle(w190) -> ("Desc"=w189:string, "TipStrip"=w188:string, "Label.Text"=w187:string, "Label.Visible"=w186:bool, "Caption.Text"=w185:string, "Caption.Visible"=w184:bool, "Disabled"=w183:u8)
            n123 = property class="Ctl"(reference=w182, "Desc"=w189, "TipStrip"=w188, "Label.Text"=w187, "Label.Visible"=w186, "Caption.Text"=w185, "Caption.Visible"=w184, "Disabled"=w183) -> ()  [unwired: 1 in, 2 out]
          }
        }
      }
      event "Help": Value Change {
        n124 = event-data() -> ()  [unwired: 1 in, 6 out]
        n125 = Control Online Help(2:path "<helpdir>/sndvibtk.chm" ("Path to the help file"), 3:"Shaft_Centerline_DB.html" ("String to search for"), 4:enum16{"Contents", "Key", "Close"}."Key" ("Operation")) -> ()  [unwired: 1 in, 1 out]
      }
      event "Label.Visible": Value Change {
        n126 = event-data() -> ("NewVal"=w197:bool)  [unwired: 1 in]
        n127 = property class="Ctl"(reference=w200, "Label.Visible"=w197) -> ()  [unwired: 1 in, 2 out]
        n128 = Select(t=u8 0 ("Disabled"), s=w197, f=u8 2) -> (s? t:f=w196:u8)
        n129 = property on="Label.Text" class="Str"("Disabled"=w196) -> ()  [unwired: 2 in, 2 out]
      }
      event "Caption.Visible": Value Change {
        n130 = event-data() -> ("NewVal"=w203:bool)  [unwired: 1 in]
        n131 = property class="Ctl"(reference=w206, "Caption.Visible"=w203) -> ()  [unwired: 1 in, 2 out]
        n132 = Select(t=u8 0 ("Disabled"), s=w203, f=u8 2) -> (s? t:f=w202:u8)
        n133 = property on="Caption.Text" class="Str"("Disabled"=w202) -> ()  [unwired: 2 in, 2 out]
      }
      event "Label.Text": Value Change {
        n134 = event-data() -> ("NewVal"=w208:string)  [unwired: 1 in]
        n135 = property class="Ctl"(reference=w209, "Label.Text"=w208) -> ()  [unwired: 1 in, 2 out]
      }
      event "Caption.Text": Value Change {
        n136 = event-data() -> ("NewVal"=w211:string)  [unwired: 1 in]
        n137 = property class="Ctl"(reference=w212, "Caption.Text"=w211) -> ()  [unwired: 1 in, 2 out]
      }
      event "Enable State": Value Change {
        n138 = event-data() -> ("NewVal"=w214:T8)  [unwired: 1 in]
        n139 = property class="Ctl"(reference=w215, "Disabled"=w214) -> ()  [unwired: 1 in, 2 out]
      }
      event "Background.Color": Value Change {
        w216 = T17[] [enum."[Plot] Grid&BG"] items=["None", "[Axis] Autoscale", "[Image] Update", "[Cursor] Name", "[Plot] Grid&BG", "[Marker] Update", "[Tree] Tags", "[Data] Update", "[Layout] Size", "[Tree] Checkbox", "[Tree] Visible", "[Tree] Open", "[Axis] X", "[Axis] Y", "[Plot] Color", "[Axis] Format String", "[Data] Compare Strings", "[Cursor] Apearance", "[Axis] Name&Visible", "[Tree] Color", "[Data] Index", "[Cursor] Index", "[Axis] Event"]
        n140 = event-data() -> ("NewVal"=w217:u32)  [unwired: 1 in]
        n141 = Bundle By Name(cluster=w219, "Background color"=w217) -> (w218:T2)
      }
      event "Legend Background.Color": Value Change {
        w220 = T17[] [enum."[Tree] Color"] items=["None", "[Axis] Autoscale", "[Image] Update", "[Cursor] Name", "[Plot] Grid&BG", "[Marker] Update", "[Tree] Tags", "[Data] Update", "[Layout] Size", "[Tree] Checkbox", "[Tree] Visible", "[Tree] Open", "[Axis] X", "[Axis] Y", "[Plot] Color", "[Axis] Format String", "[Data] Compare Strings", "[Cursor] Apearance", "[Axis] Name&Visible", "[Tree] Color", "[Data] Index", "[Cursor] Index", "[Axis] Event"]
        n142 = event-data() -> ("NewVal"=w221:u32)  [unwired: 1 in]
        n143 = Bundle By Name(cluster=w223, "Legend Background"=w221) -> (w222:T2)
      }
      event "Legend Font.Color": Value Change {
        w224 = T17[] [enum."[Tree] Color"] items=["None", "[Axis] Autoscale", "[Image] Update", "[Cursor] Name", "[Plot] Grid&BG", "[Marker] Update", "[Tree] Tags", "[Data] Update", "[Layout] Size", "[Tree] Checkbox", "[Tree] Visible", "[Tree] Open", "[Axis] X", "[Axis] Y", "[Plot] Color", "[Axis] Format String", "[Data] Compare Strings", "[Cursor] Apearance", "[Axis] Name&Visible", "[Tree] Color", "[Data] Index", "[Cursor] Index", "[Axis] Event"]
        n144 = event-data() -> ("NewVal"=w225:u32)  [unwired: 1 in]
        n145 = Bundle By Name(cluster=w227, "Legend Font"=w225) -> (w226:T2)
      }
      event "Direction.Color", "Clearance Boundary.Color": Value Change {
        w228 = T17[] [enum."[Image] Update"] items=["None", "[Axis] Autoscale", "[Image] Update", "[Cursor] Name", "[Plot] Grid&BG", "[Marker] Update", "[Tree] Tags", "[Data] Update", "[Layout] Size", "[Tree] Checkbox", "[Tree] Visible", "[Tree] Open", "[Axis] X", "[Axis] Y", "[Plot] Color", "[Axis] Format String", "[Data] Compare Strings", "[Cursor] Apearance", "[Axis] Name&Visible", "[Tree] Color", "[Data] Index", "[Cursor] Index", "[Axis] Event"]
        n146 = event-data() -> ()  [unwired: 1 in, 1 out]
        n147 = Bundle By Name(cluster=w229, "Arrow Color"="Direction.Color", "Boundary Color"="Clearance Boundary.Color") -> (w232:T2)
      }
      event "Digits", "Hide trailing zeros", "Type", "Precision Type": Value Change {
        w233 = T17[] [enum."[Axis] Format String"] items=["None", "[Axis] Autoscale", "[Image] Update", "[Cursor] Name", "[Plot] Grid&BG", "[Marker] Update", "[Tree] Tags", "[Data] Update", "[Layout] Size", "[Tree] Checkbox", "[Tree] Visible", "[Tree] Open", "[Axis] X", "[Axis] Y", "[Plot] Color", "[Axis] Format String", "[Data] Compare Strings", "[Cursor] Apearance", "[Axis] Name&Visible", "[Tree] Color", "[Data] Index", "[Cursor] Index", "[Axis] Event"]
        n148 = event-data() -> ()  [unwired: 1 in, 1 out]
        n149 = call <vilib>:"svx_SC Line To FString.vi"("trailing zeros"="Hide trailing zeros", "Precision Type"="Precision Type", "Digits"="Digits", "Type"="Type") -> ("format string"=w236:string)  [unwired: 7 in]
        n150 = case shown="0, Default" "Format Selection" {
          tunnel: w236 -> [w242 w245]
          tunnel: w235 -> [w244 w247]
          tunnel: [w243 w246] -> w234
          frame 0, Default {
            n151 = Bundle By Name(cluster=w244, "X Scale.format string"=w242) -> (w243:T2)
          }
          frame 1 {
            n152 = Bundle By Name(cluster=w247, "Y Scale.format string"=w245) -> (w246:T2)
          }
        }
      }
      event "Format Selection": Value Change {
        n153 = event-data() -> ("NewVal"=w254:u16)  [unwired: 1 in]
        n154 = case shown="1" w254 {
          tunnel: w253 -> [w256 w258]
          tunnel: [w255 w257] -> w252
          frame 0, Default {
            n155 = Unbundle By Name(w256) -> ("X Scale.format string"=w255:string)
          }
          frame 1 {
            n156 = Unbundle By Name(w258) -> ("Y Scale.format string"=w257:string)
          }
        }
        n157 = call <vilib>:"svx_SC Line From FString.vi"("Format string"=w252) -> ("trailing zeros"=w248:bool, "Precision Type"=w249:u16, "Digits"=w250:u8, "Type"=w251:i32)  [unwired: 7 in]
        n158 = local write "Hide trailing zeros"(w248) -> ()
        n159 = local write "Precision Type"(w249) -> ()
        n160 = local write "Digits"(w250) -> ()
        n161 = local write "Type"(w251) -> ()
      }
      event "Plot.Line Style": Value Change {
        w259 = T17[] [enum."[Plot] Color"] items=["None", "[Axis] Autoscale", "[Image] Update", "[Cursor] Name", "[Plot] Grid&BG", "[Marker] Update", "[Tree] Tags", "[Data] Update", "[Layout] Size", "[Tree] Checkbox", "[Tree] Visible", "[Tree] Open", "[Axis] X", "[Axis] Y", "[Plot] Color", "[Axis] Format String", "[Data] Compare Strings", "[Cursor] Apearance", "[Axis] Name&Visible", "[Tree] Color", "[Data] Index", "[Cursor] Index", "[Axis] Event"]
        w268 = bool[] []
        n162 = event-data() -> ("CtlRef"=w263:refnum<vi>, "OldVal"=w269:T10, "NewVal"=w270:T10)  [unwired: 1 in]
        n163 = Variant To Data(type=w268, Variant=w270) -> (data=w267:bool[])  [unwired: 1 in, 1 out]
        n164 = Variant To Data(type=w268, Variant=w269) -> (data=w266:bool[])  [unwired: 1 in, 1 out]
        n165 = Exclusive Or(1:w267, 2:w266) -> (0:w265:bool[])
        n166 = Search 1D Array(1D array=w265, element=TRUE) -> (index of element=w260:i32)  [unwired: 1 in]
        n167 = Bundle By Name(cluster=w262, "Plot.Line Style"=w260) -> (w261:T2)
        n168 = call <vilib>:"svx_SC Line Manage Cluster.vi"("index"=w260, "Clust Refnum"=w263) -> ()  [unwired: 10 in]
      }
      event "Plot.Line Width": Value Change {
        w271 = T17[] [enum."[Plot] Color"] items=["None", "[Axis] Autoscale", "[Image] Update", "[Cursor] Name", "[Plot] Grid&BG", "[Marker] Update", "[Tree] Tags", "[Data] Update", "[Layout] Size", "[Tree] Checkbox", "[Tree] Visible", "[Tree] Open", "[Axis] X", "[Axis] Y", "[Plot] Color", "[Axis] Format String", "[Data] Compare Strings", "[Cursor] Apearance", "[Axis] Name&Visible", "[Tree] Color", "[Data] Index", "[Cursor] Index", "[Axis] Event"]
        w282 = bool[] []
        n169 = event-data() -> ("CtlRef"=w272:refnum<vi>, "OldVal"=w273:T11, "NewVal"=w274:T11)  [unwired: 1 in]
        n170 = Variant To Data(type=w282, Variant=w274) -> (data=w281:bool[])  [unwired: 1 in, 1 out]
        n171 = Variant To Data(type=w282, Variant=w273) -> (data=w280:bool[])  [unwired: 1 in, 1 out]
        n172 = Exclusive Or(1:w281, 2:w280) -> (0:w279:bool[])
        n173 = Search 1D Array(1D array=w279, element=TRUE) -> (index of element=w275:i32)  [unwired: 1 in]
        n174 = Bundle By Name(cluster=w277, "Plot.Line Width"=w275) -> (w276:T2)
        n175 = call <vilib>:"svx_SC Line Manage Cluster.vi"("index"=w275, "Clust Refnum"=w272) -> ()  [unwired: 10 in]
      }
      event "Plot.Point Style": Value Change {
        w283 = T17[] [enum."[Plot] Color"] items=["None", "[Axis] Autoscale", "[Image] Update", "[Cursor] Name", "[Plot] Grid&BG", "[Marker] Update", "[Tree] Tags", "[Data] Update", "[Layout] Size", "[Tree] Checkbox", "[Tree] Visible", "[Tree] Open", "[Axis] X", "[Axis] Y", "[Plot] Color", "[Axis] Format String", "[Data] Compare Strings", "[Cursor] Apearance", "[Axis] Name&Visible", "[Tree] Color", "[Data] Index", "[Cursor] Index", "[Axis] Event"]
        w294 = bool[] []
        n176 = event-data() -> ("CtlRef"=w284:refnum<vi>, "OldVal"=w285:T9, "NewVal"=w286:T9)  [unwired: 1 in]
        n177 = Variant To Data(type=w294, Variant=w286) -> (data=w293:bool[])  [unwired: 1 in, 1 out]
        n178 = Variant To Data(type=w294, Variant=w285) -> (data=w292:bool[])  [unwired: 1 in, 1 out]
        n179 = Exclusive Or(1:w293, 2:w292) -> (0:w291:bool[])
        n180 = Search 1D Array(1D array=w291, element=TRUE) -> (index of element=w287:i32)  [unwired: 1 in]
        n181 = Bundle By Name(cluster=w289, "Plot.Point Style"=w287) -> (w288:T2)
        n182 = call <vilib>:"svx_SC Line Manage Cluster.vi"("index"=w287, "Clust Refnum"=w284) -> ()  [unwired: 10 in]
      }
      event "Line.Color": Value Change {
        w295 = T17[] [enum."[Plot] Color"] items=["None", "[Axis] Autoscale", "[Image] Update", "[Cursor] Name", "[Plot] Grid&BG", "[Marker] Update", "[Tree] Tags", "[Data] Update", "[Layout] Size", "[Tree] Checkbox", "[Tree] Visible", "[Tree] Open", "[Axis] X", "[Axis] Y", "[Plot] Color", "[Axis] Format String", "[Data] Compare Strings", "[Cursor] Apearance", "[Axis] Name&Visible", "[Tree] Color", "[Data] Index", "[Cursor] Index", "[Axis] Event"]
        n183 = event-data() -> ("NewVal"=w296:u32)  [unwired: 1 in]
        n184 = Bundle By Name(cluster=w298, "Plot.Plot Color"=w296) -> (w297:T2)
      }
      event "Point/Fill.Color": Value Change {
        w299 = T17[] [enum."[Plot] Color"] items=["None", "[Axis] Autoscale", "[Image] Update", "[Cursor] Name", "[Plot] Grid&BG", "[Marker] Update", "[Tree] Tags", "[Data] Update", "[Layout] Size", "[Tree] Checkbox", "[Tree] Visible", "[Tree] Open", "[Axis] X", "[Axis] Y", "[Plot] Color", "[Axis] Format String", "[Data] Compare Strings", "[Cursor] Apearance", "[Axis] Name&Visible", "[Tree] Color", "[Data] Index", "[Cursor] Index", "[Axis] Event"]
        n185 = event-data() -> ("NewVal"=w300:u32)  [unwired: 1 in]
        n186 = Bundle By Name(cluster=w302, "Plot.Point/fill"=w300) -> (w301:T2)
      }
      event "Scale Name": Value Change {
        w303 = T17[] [enum."[Axis] Name&Visible"] items=["None", "[Axis] Autoscale", "[Image] Update", "[Cursor] Name", "[Plot] Grid&BG", "[Marker] Update", "[Tree] Tags", "[Data] Update", "[Layout] Size", "[Tree] Checkbox", "[Tree] Visible", "[Tree] Open", "[Axis] X", "[Axis] Y", "[Plot] Color", "[Axis] Format String", "[Data] Compare Strings", "[Cursor] Apearance", "[Axis] Name&Visible", "[Tree] Color", "[Data] Index", "[Cursor] Index", "[Axis] Event"]
        n187 = event-data() -> ("NewVal"=w307:string)  [unwired: 1 in]
        n188 = local read "Scale Selection"() -> (w309:u16)
        n189 = property on="Scale Selection" class="Ring (strict)"() -> ("Strings []"=w308:string[])  [unwired: 2 in, 2 out]
        n190 = case shown="1" w309 {
          tunnel: w307 -> [w313 w317]
          tunnel: w311 -> [w315 w319]
          tunnel: [w314 w318] -> w310
          tunnel: [" (X-Axis)" ("string") " (Y-Axis)" ("string")] -> w304
          frame 0, Default {
            n191 = Bundle By Name(cluster=w315, "X Scale.Name"=w313) -> (w314:T2)
          }
          frame 1 {
            n192 = Bundle By Name(cluster=w319, "Y Scale.Name"=w317) -> (w318:T2)
          }
        }
        n193 = Concatenate Strings(w307, w304) -> (w306:string)
        n194 = Replace Array Subset(array=w308, new element=w306, index=w309) -> (w305:string[])
        n195 = property on="Scale Selection" class="Ring (strict)"("Strings []"=w305) -> ()  [unwired: 2 in, 2 out]
        n196 = property on="Format Selection" class="Ring (strict)"("Strings []"=w305) -> ()  [unwired: 2 in, 2 out]
      }
      event "Scale Label.Visible": Value Change {
        w320 = T17[] [enum."[Axis] Name&Visible"] items=["None", "[Axis] Autoscale", "[Image] Update", "[Cursor] Name", "[Plot] Grid&BG", "[Marker] Update", "[Tree] Tags", "[Data] Update", "[Layout] Size", "[Tree] Checkbox", "[Tree] Visible", "[Tree] Open", "[Axis] X", "[Axis] Y", "[Plot] Color", "[Axis] Format String", "[Data] Compare Strings", "[Cursor] Apearance", "[Axis] Name&Visible", "[Tree] Color", "[Data] Index", "[Cursor] Index", "[Axis] Event"]
        n197 = event-data() -> ("NewVal"=w322:bool)  [unwired: 1 in]
        n198 = local read "Scale Selection"() -> (w321:u16)
        n199 = case shown="1" w321 {
          tunnel: w322 -> [w325 w328]
          tunnel: w324 -> [w327 w330]
          tunnel: [w326 w329] -> w323
          frame 0, Default {
            n200 = Bundle By Name(cluster=w327, "X Scale.Label Visible"=w325) -> (w326:T2)
          }
          frame 1 {
            n201 = Bundle By Name(cluster=w330, "Y Scale.Label Visible"=w328) -> (w329:T2)
          }
        }
      }
      event "Scale.Visible": Value Change {
        w331 = T17[] [enum."[Axis] Name&Visible"] items=["None", "[Axis] Autoscale", "[Image] Update", "[Cursor] Name", "[Plot] Grid&BG", "[Marker] Update", "[Tree] Tags", "[Data] Update", "[Layout] Size", "[Tree] Checkbox", "[Tree] Visible", "[Tree] Open", "[Axis] X", "[Axis] Y", "[Plot] Color", "[Axis] Format String", "[Data] Compare Strings", "[Cursor] Apearance", "[Axis] Name&Visible", "[Tree] Color", "[Data] Index", "[Cursor] Index", "[Axis] Event"]
        n202 = event-data() -> ("NewVal"=w333:bool)  [unwired: 1 in]
        n203 = local read "Scale Selection"() -> (w332:u16)
        n204 = case shown="1" w332 {
          tunnel: w333 -> [w336 w339]
          tunnel: w335 -> [w338 w341]
          tunnel: [w337 w340] -> w334
          frame 0, Default {
            n205 = Bundle By Name(cluster=w338, "X Scale.Scale Visible"=w336) -> (w337:T2)
          }
          frame 1 {
            n206 = Bundle By Name(cluster=w341, "Y Scale.Scale Visible"=w339) -> (w340:T2)
          }
        }
      }
      event "Scale Fit": Value Change {
        w348 = T17[] [enum."[Marker] Update", enum."[Image] Update"] items=["None", "[Axis] Autoscale", "[Image] Update", "[Cursor] Name", "[Plot] Grid&BG", "[Marker] Update", "[Tree] Tags", "[Data] Update", "[Layout] Size", "[Tree] Checkbox", "[Tree] Visible", "[Tree] Open", "[Axis] X", "[Axis] Y", "[Plot] Color", "[Axis] Format String", "[Data] Compare Strings", "[Cursor] Apearance", "[Axis] Name&Visible", "[Tree] Color", "[Data] Index", "[Cursor] Index", "[Axis] Event"]
        n207 = event-data() -> ("NewVal"=w345:bool)  [unwired: 1 in]
        n208 = Boolean To (0,1)(Boolean=w345) -> (0, 1=w353:i16)
        n209 = Add(x=w353, y=w353) -> (x+y=w346:i16)
        n210 = Select(t=u8 2 ("scale fit"), s=w345, f=u8 0 ("scale fit")) -> (s? t:f=w342:u8)
        n211 = local read "Scale Selection"() -> (w352:u16)
        n212 = property on="Minimum" class="DigNum (strict)"("Disabled"=w346) -> ()  [unwired: 2 in, 2 out]
        n213 = property on="Maximum" class="DigNum (strict)"("Disabled"=w346) -> ()  [unwired: 2 in, 2 out]
        n214 = Bundle By Name(cluster=w351, "Autoscale"=w345, "scale fit"=w342) -> (w350:T2)
        n215 = call <vilib>:"svx_SC Line Autoscale.vi"("State In"=w350, "SC Line in"=w349) -> ("State Out"=w347:T2)  [unwired: 7 in, 2 out]
        n216 = case shown="True" w345 {
          tunnel: w347 -> [_ w356]
          tunnel: w352 -> [_ w357]
          frame False {
          }
          frame True {
            n217 = case shown="1" w357 {
              tunnel: w356 -> [w360 w363]
              tunnel: [w359 w362] -> w355
              tunnel: [w358 w361] -> w354
              frame 0, Default {
                n218 = Unbundle By Name(w360) -> ("X Scale.Maximum"=w359:dbl, "X Scale.Minimum"=w358:dbl)
              }
              frame 1 {
                n219 = Unbundle By Name(w363) -> ("Y Scale.Maximum"=w362:dbl, "Y Scale.Minimum"=w361:dbl)
              }
            }
            n220 = local write "Minimum"(w354) -> ()
            n221 = local write "Maximum"(w355) -> ()
          }
        }
      }
      event "Maximum", "Minimum": Value Change {
        n222 = event-data() -> ("NewVal"=w368:dbl)  [unwired: 1 in]
        n223 = local read "Scale Selection"() -> (w367:u16)
        n224 = case shown="1" w367 {
          tunnel: w368 -> [w374 _]
          tunnel: w366 -> [w373 w378]
          tunnel: [w370 w375] -> w365
          tunnel: [w369 w379] -> w364
          frame 0, Default {
            w369 = T17[] [enum."[Axis] X"] items=["None", "[Axis] Autoscale", "[Image] Update", "[Cursor] Name", "[Plot] Grid&BG", "[Marker] Update", "[Tree] Tags", "[Data] Update", "[Layout] Size", "[Tree] Checkbox", "[Tree] Visible", "[Tree] Open", "[Axis] X", "[Axis] Y", "[Plot] Color", "[Axis] Format String", "[Data] Compare Strings", "[Cursor] Apearance", "[Axis] Name&Visible", "[Tree] Color", "[Data] Index", "[Cursor] Index", "[Axis] Event"]
            n225 = Absolute Value(x=w374) -> (abs(x)=w371:dbl)
            n226 = Negate(x=w371) -> (-x=w372:dbl)
            n227 = local write "Minimum"(w372) -> ()
            n228 = local write "Maximum"(w371) -> ()
            n229 = Bundle By Name(cluster=w373, "X Scale.Minimum"=w372, "X Scale.Maximum"=w371) -> (w370:T2)
          }
          frame 1 {
            w379 = T17[] [enum."[Axis] Y"] items=["None", "[Axis] Autoscale", "[Image] Update", "[Cursor] Name", "[Plot] Grid&BG", "[Marker] Update", "[Tree] Tags", "[Data] Update", "[Layout] Size", "[Tree] Checkbox", "[Tree] Visible", "[Tree] Open", "[Axis] X", "[Axis] Y", "[Plot] Color", "[Axis] Format String", "[Data] Compare Strings", "[Cursor] Apearance", "[Axis] Name&Visible", "[Tree] Color", "[Data] Index", "[Cursor] Index", "[Axis] Event"]
            n230 = local read "Minimum"() -> (w381:dbl)
            n231 = local read "Maximum"() -> (w380:dbl)
            n232 = Max & Min(x=w381, y=w380) -> (max(x,y)=w377:dbl, min(x,y)=w376:dbl)
            n233 = local write "Minimum"(w376) -> ()
            n234 = local write "Maximum"(w377) -> ()
            n235 = Bundle By Name(cluster=w378, "Y Scale.Maximum"=w377, "Y Scale.Minimum"=w376) -> (w375:T2)
          }
        }
      }
      event "XGrid Style": Value Change {
        w382 = T17[] [enum."[Plot] Grid&BG"] items=["None", "[Axis] Autoscale", "[Image] Update", "[Cursor] Name", "[Plot] Grid&BG", "[Marker] Update", "[Tree] Tags", "[Data] Update", "[Layout] Size", "[Tree] Checkbox", "[Tree] Visible", "[Tree] Open", "[Axis] X", "[Axis] Y", "[Plot] Color", "[Axis] Format String", "[Data] Compare Strings", "[Cursor] Apearance", "[Axis] Name&Visible", "[Tree] Color", "[Data] Index", "[Cursor] Index", "[Axis] Event"]
        n236 = event-data() -> ("NewVal"=w385:u16)  [unwired: 1 in]
        n237 = Bundle By Name(cluster=w386, "X Scale.Grid Style"=w385) -> (w387:T2)
        n238 = case shown="1" w385 {
          tunnel: [w388 u8 0 ("Disabled") w391] -> w384
          tunnel: [w388 u8 2 ("Disabled") w391] -> w383
          frame 0, Default {
            w388 = u8 2 ("Disabled")
          }
          frame 1 {
          }
          frame 2 {
            w391 = u8 0 ("Disabled")
          }
        }
        n239 = property on="Major Grid.Color" class="ColBox"("Disabled"=w384) -> ()  [unwired: 2 in, 2 out]
        n240 = property on="Minor Grid.Color" class="ColBox"("Disabled"=w383) -> ()  [unwired: 2 in, 2 out]
      }
      event "YGrid Style": Value Change {
        w392 = T17[] [enum."[Plot] Grid&BG"] items=["None", "[Axis] Autoscale", "[Image] Update", "[Cursor] Name", "[Plot] Grid&BG", "[Marker] Update", "[Tree] Tags", "[Data] Update", "[Layout] Size", "[Tree] Checkbox", "[Tree] Visible", "[Tree] Open", "[Axis] X", "[Axis] Y", "[Plot] Color", "[Axis] Format String", "[Data] Compare Strings", "[Cursor] Apearance", "[Axis] Name&Visible", "[Tree] Color", "[Data] Index", "[Cursor] Index", "[Axis] Event"]
        n241 = event-data() -> ("NewVal"=w395:u16)  [unwired: 1 in]
        n242 = case shown="1" w395 {
          tunnel: [w398 u8 0 ("Disabled") w401] -> w394
          tunnel: [w398 u8 2 ("Disabled") w401] -> w393
          frame 0, Default {
            w398 = u8 2 ("Disabled")
          }
          frame 1 {
          }
          frame 2 {
            w401 = u8 0 ("Disabled")
          }
        }
        n243 = Bundle By Name(cluster=w396, "Y Scale.Grid Style"=w395) -> (w397:T2)
        n244 = property on="Major Grid.Color" class="ColBox"("Disabled"=w394) -> ()  [unwired: 2 in, 2 out]
        n245 = property on="Minor Grid.Color" class="ColBox"("Disabled"=w393) -> ()  [unwired: 2 in, 2 out]
      }
      event "Major Grid.Color": Value Change {
        w402 = T17[] [enum."[Plot] Grid&BG"] items=["None", "[Axis] Autoscale", "[Image] Update", "[Cursor] Name", "[Plot] Grid&BG", "[Marker] Update", "[Tree] Tags", "[Data] Update", "[Layout] Size", "[Tree] Checkbox", "[Tree] Visible", "[Tree] Open", "[Axis] X", "[Axis] Y", "[Plot] Color", "[Axis] Format String", "[Data] Compare Strings", "[Cursor] Apearance", "[Axis] Name&Visible", "[Tree] Color", "[Data] Index", "[Cursor] Index", "[Axis] Event"]
        n246 = event-data() -> ("NewVal"=w404:u32)  [unwired: 1 in]
        n247 = local read "Scale Selection"() -> (w403:u16)
        n248 = case shown="1" w403 {
          tunnel: w406 -> [w409 w412]
          tunnel: [w408 w411] -> w405
          tunnel: w404 -> [w407 w410]
          frame 0, Default {
            n249 = Bundle By Name(cluster=w409, "X Scale.Major Color"=w407) -> (w408:T2)
          }
          frame 1 {
            n250 = Bundle By Name(cluster=w412, "Y Scale.Major Color"=w410) -> (w411:T2)
          }
        }
      }
      event "Minor Grid.Color": Value Change {
        w413 = T17[] [enum."[Plot] Grid&BG"] items=["None", "[Axis] Autoscale", "[Image] Update", "[Cursor] Name", "[Plot] Grid&BG", "[Marker] Update", "[Tree] Tags", "[Data] Update", "[Layout] Size", "[Tree] Checkbox", "[Tree] Visible", "[Tree] Open", "[Axis] X", "[Axis] Y", "[Plot] Color", "[Axis] Format String", "[Data] Compare Strings", "[Cursor] Apearance", "[Axis] Name&Visible", "[Tree] Color", "[Data] Index", "[Cursor] Index", "[Axis] Event"]
        n251 = event-data() -> ("NewVal"=w415:u32)  [unwired: 1 in]
        n252 = local read "Scale Selection"() -> (w414:u16)
        n253 = case shown="0, Default" w414 {
          tunnel: w417 -> [w420 w423]
          tunnel: [w419 w422] -> w416
          tunnel: w415 -> [w418 w421]
          frame 0, Default {
            n254 = Bundle By Name(cluster=w420, "X Scale.Minor Color"=w418) -> (w419:T2)
          }
          frame 1 {
            n255 = Bundle By Name(cluster=w423, "Y Scale.Minor Color"=w421) -> (w422:T2)
          }
        }
      }
      event "Scale Selection": Value Change {
        n256 = event-data() -> ("NewVal"=w428:u16)  [unwired: 1 in]
        n257 = case shown="1" w428 {
          tunnel: [w451 w463] -> w436
          tunnel: [w450 w462] -> w433
          tunnel: [w449 w461] -> w432
          tunnel: [w448 w460] -> w431
          tunnel: [w447 w459] -> w430
          tunnel: [w446 w458] -> w429
          tunnel: w427 -> [w445 w457]
          tunnel: [w442 w454] -> w426
          tunnel: [w441 w453] -> w425
          tunnel: [w440 w452] -> w424
          frame 0, Default {
            n258 = Unbundle By Name(w445) -> ("X Scale.Name"=w446:string, "X Scale.Label Visible"=w447:bool, "X Scale.Scale Visible"=w448:bool, "X Scale.Major Color"=w449:u32, "X Scale.Minor Color"=w450:u32, "Autoscale"=w451:bool, "X Scale.Minimum"=w441:dbl, "X Scale.Maximum"=w440:dbl, "X Scale.Grid Style"=w442:u16)
            n259 = property on="XGrid Style" class="Ring (strict)"("Visible"=TRUE) -> ()  [unwired: 2 in, 2 out]
            n260 = local write "XGrid Style"(w442) -> ()
            n261 = property on="YGrid Style" class="Ring (strict)"("Visible"=FALSE) -> ()  [unwired: 2 in, 2 out]
          }
          frame 1 {
            n262 = Unbundle By Name(w457) -> ("Y Scale.Name"=w458:string, "Y Scale.Label Visible"=w459:bool, "Y Scale.Scale Visible"=w460:bool, "Y Scale.Major Color"=w461:u32, "Y Scale.Minor Color"=w462:u32, "Autoscale"=w463:bool, "Y Scale.Minimum"=w453:dbl, "Y Scale.Maximum"=w452:dbl, "Y Scale.Grid Style"=w454:u16)
            n263 = property on="XGrid Style" class="Ring (strict)"("Visible"=FALSE) -> ()  [unwired: 2 in, 2 out]
            n264 = local write "YGrid Style"(w454) -> ()
            n265 = property on="YGrid Style" class="Ring (strict)"("Visible"=TRUE) -> ()  [unwired: 2 in, 2 out]
          }
        }
        n266 = local write "Minimum"(w425) -> ()
        n267 = local write "Maximum"(w424) -> ()
        n268 = local write "Scale Name"(w429) -> ()
        n269 = local write "Scale.Visible"(w431) -> ()
        n270 = local write "Minor Grid.Color"(w433) -> ()
        n271 = case shown="2" w426 {
          tunnel: [w464 u8 0 ("Disabled") w467] -> w438
          tunnel: [w464 u8 2 ("Disabled") w467] -> w439
          frame 0, Default {
            w464 = u8 2 ("Disabled")
          }
          frame 1 {
          }
          frame 2 {
            w467 = u8 0 ("Disabled")
          }
        }
        n272 = Select(t=u8 2 ("Disabled"), s=w436, f=u8 0) -> (s? t:f=w437:u8)
        n273 = local write "Scale Label.Visible"(w430) -> ()
        n274 = local write "Major Grid.Color"(w432) -> ()
        n275 = local write "Scale Fit"(w436) -> ()
        n276 = property on="Minimum" class="DigNum (strict)"("Disabled"=w437) -> ()  [unwired: 2 in, 2 out]
        n277 = property on="Maximum" class="DigNum (strict)"("Disabled"=w437) -> ()  [unwired: 2 in, 2 out]
        n278 = property on="Major Grid.Color" class="ColBox"("Disabled"=w438) -> ()  [unwired: 2 in, 2 out]
        n279 = property on="Minor Grid.Color" class="ColBox"("Disabled"=w439) -> ()  [unwired: 2 in, 2 out]
      }
      event "Cursor.Line Style": Value Change {
        w468 = T17[] [enum."[Cursor] Apearance"] items=["None", "[Axis] Autoscale", "[Image] Update", "[Cursor] Name", "[Plot] Grid&BG", "[Marker] Update", "[Tree] Tags", "[Data] Update", "[Layout] Size", "[Tree] Checkbox", "[Tree] Visible", "[Tree] Open", "[Axis] X", "[Axis] Y", "[Plot] Color", "[Axis] Format String", "[Data] Compare Strings", "[Cursor] Apearance", "[Axis] Name&Visible", "[Tree] Color", "[Data] Index", "[Cursor] Index", "[Axis] Event"]
        w479 = bool[] []
        n280 = event-data() -> ("CtlRef"=w469:refnum<vi>, "OldVal"=w470:T10, "NewVal"=w471:T10)  [unwired: 1 in]
        n281 = Variant To Data(type=w479, Variant=w471) -> (data=w478:bool[])  [unwired: 1 in, 1 out]
        n282 = Variant To Data(type=w479, Variant=w470) -> (data=w477:bool[])  [unwired: 1 in, 1 out]
        n283 = Exclusive Or(1:w478, 2:w477) -> (0:w476:bool[])
        n284 = Search 1D Array(1D array=w476, element=TRUE) -> (index of element=w472:i32)  [unwired: 1 in]
        n285 = Bundle By Name(cluster=w474, "Cursor.Cursor Line Style"=w472) -> (w473:T2)
        n286 = call <vilib>:"svx_SC Line Manage Cluster.vi"("index"=w472, "Clust Refnum"=w469) -> ()  [unwired: 10 in]
      }
      event "Cursor.Line Width": Value Change {
        w480 = T17[] [enum."[Cursor] Apearance"] items=["None", "[Axis] Autoscale", "[Image] Update", "[Cursor] Name", "[Plot] Grid&BG", "[Marker] Update", "[Tree] Tags", "[Data] Update", "[Layout] Size", "[Tree] Checkbox", "[Tree] Visible", "[Tree] Open", "[Axis] X", "[Axis] Y", "[Plot] Color", "[Axis] Format String", "[Data] Compare Strings", "[Cursor] Apearance", "[Axis] Name&Visible", "[Tree] Color", "[Data] Index", "[Cursor] Index", "[Axis] Event"]
        w491 = bool[] []
        n287 = event-data() -> ("CtlRef"=w481:refnum<vi>, "OldVal"=w482:T11, "NewVal"=w483:T11)  [unwired: 1 in]
        n288 = Variant To Data(type=w491, Variant=w483) -> (data=w490:bool[])  [unwired: 1 in, 1 out]
        n289 = Variant To Data(type=w491, Variant=w482) -> (data=w489:bool[])  [unwired: 1 in, 1 out]
        n290 = Exclusive Or(1:w490, 2:w489) -> (0:w488:bool[])
        n291 = Search 1D Array(1D array=w488, element=TRUE) -> (index of element=w484:i32)  [unwired: 1 in]
        n292 = Bundle By Name(cluster=w486, "Cursor.Cursor Line Width"=w484) -> (w485:T2)
        n293 = call <vilib>:"svx_SC Line Manage Cluster.vi"("index"=w484, "Clust Refnum"=w481) -> ()  [unwired: 10 in]
      }
      event "Cursor.Point Style": Value Change {
        w492 = T17[] [enum."[Cursor] Apearance"] items=["None", "[Axis] Autoscale", "[Image] Update", "[Cursor] Name", "[Plot] Grid&BG", "[Marker] Update", "[Tree] Tags", "[Data] Update", "[Layout] Size", "[Tree] Checkbox", "[Tree] Visible", "[Tree] Open", "[Axis] X", "[Axis] Y", "[Plot] Color", "[Axis] Format String", "[Data] Compare Strings", "[Cursor] Apearance", "[Axis] Name&Visible", "[Tree] Color", "[Data] Index", "[Cursor] Index", "[Axis] Event"]
        w503 = bool[] []
        n294 = event-data() -> ("CtlRef"=w493:refnum<vi>, "OldVal"=w494:T9, "NewVal"=w495:T9)  [unwired: 1 in]
        n295 = Variant To Data(type=w503, Variant=w495) -> (data=w502:bool[])  [unwired: 1 in, 1 out]
        n296 = Variant To Data(type=w503, Variant=w494) -> (data=w501:bool[])  [unwired: 1 in, 1 out]
        n297 = Exclusive Or(1:w502, 2:w501) -> (0:w500:bool[])
        n298 = Search 1D Array(1D array=w500, element=TRUE) -> (index of element=w496:i32)  [unwired: 1 in]
        n299 = Bundle By Name(cluster=w498, "Cursor.Cursor Point Style"=w496) -> (w497:T2)
        n300 = call <vilib>:"svx_SC Line Manage Cluster.vi"("index"=w496, "Clust Refnum"=w493) -> ()  [unwired: 10 in]
      }
      event "Cursor.Style": Value Change {
        w504 = T17[] [enum."[Cursor] Apearance"] items=["None", "[Axis] Autoscale", "[Image] Update", "[Cursor] Name", "[Plot] Grid&BG", "[Marker] Update", "[Tree] Tags", "[Data] Update", "[Layout] Size", "[Tree] Checkbox", "[Tree] Visible", "[Tree] Open", "[Axis] X", "[Axis] Y", "[Plot] Color", "[Axis] Format String", "[Data] Compare Strings", "[Cursor] Apearance", "[Axis] Name&Visible", "[Tree] Color", "[Data] Index", "[Cursor] Index", "[Axis] Event"]
        w515 = bool[] []
        n301 = event-data() -> ("CtlRef"=w505:refnum<vi>, "OldVal"=w506:T12, "NewVal"=w507:T12)  [unwired: 1 in]
        n302 = Variant To Data(type=w515, Variant=w507) -> (data=w514:bool[])  [unwired: 1 in, 1 out]
        n303 = Variant To Data(type=w515, Variant=w506) -> (data=w513:bool[])  [unwired: 1 in, 1 out]
        n304 = Exclusive Or(1:w514, 2:w513) -> (0:w512:bool[])
        n305 = Search 1D Array(1D array=w512, element=TRUE) -> (index of element=w508:i32)  [unwired: 1 in]
        n306 = Bundle By Name(cluster=w510, "Cursor.Cursor Style"=w508) -> (w509:T2)
        n307 = call <vilib>:"svx_SC Line Manage Cluster.vi"("index"=w508, "Clust Refnum"=w505) -> ()  [unwired: 10 in]
      }
      event "Cursor Info.Visible": Value Change {
        w516 = T17[] [enum."[Cursor] Name"] items=["None", "[Axis] Autoscale", "[Image] Update", "[Cursor] Name", "[Plot] Grid&BG", "[Marker] Update", "[Tree] Tags", "[Data] Update", "[Layout] Size", "[Tree] Checkbox", "[Tree] Visible", "[Tree] Open", "[Axis] X", "[Axis] Y", "[Plot] Color", "[Axis] Format String", "[Data] Compare Strings", "[Cursor] Apearance", "[Axis] Name&Visible", "[Tree] Color", "[Data] Index", "[Cursor] Index", "[Axis] Event"]
        n308 = event-data() -> ("NewVal"=w517:bool)  [unwired: 1 in]
        n309 = Select(t=u8 0 ("Disabled"), s=w517, f=u8 2) -> (s? t:f=w518:u8)
        n310 = Bundle By Name(cluster=w522, "Cursor.Cursor Name Visible"=w517) -> (w521:T2)
        n311 = property on="Cursor Info Position.Lock" class="Bool (strict)"("Disabled"=w518) -> ()  [unwired: 2 in, 2 out]
      }
      event "Cursor Info Position.Lock": Value Change {
        w523 = T17[] [enum."[Cursor] Name"] items=["None", "[Axis] Autoscale", "[Image] Update", "[Cursor] Name", "[Plot] Grid&BG", "[Marker] Update", "[Tree] Tags", "[Data] Update", "[Layout] Size", "[Tree] Checkbox", "[Tree] Visible", "[Tree] Open", "[Axis] X", "[Axis] Y", "[Plot] Color", "[Axis] Format String", "[Data] Compare Strings", "[Cursor] Apearance", "[Axis] Name&Visible", "[Tree] Color", "[Data] Index", "[Cursor] Index", "[Axis] Event"]
        n312 = event-data() -> ("NewVal"=w524:bool)  [unwired: 1 in]
        n313 = Bundle By Name(cluster=w526, "Cursor.Lock Cursor Name"=w524) -> (w525:T2)
      }
      event "Cursor.Visible": Value Change {
        w527 = T17[] [enum."[Cursor] Name"] items=["None", "[Axis] Autoscale", "[Image] Update", "[Cursor] Name", "[Plot] Grid&BG", "[Marker] Update", "[Tree] Tags", "[Data] Update", "[Layout] Size", "[Tree] Checkbox", "[Tree] Visible", "[Tree] Open", "[Axis] X", "[Axis] Y", "[Plot] Color", "[Axis] Format String", "[Data] Compare Strings", "[Cursor] Apearance", "[Axis] Name&Visible", "[Tree] Color", "[Data] Index", "[Cursor] Index", "[Axis] Event"]
        n314 = event-data() -> ("NewVal"=w533:bool)  [unwired: 1 in]
        n315 = local read "Cursor Info.Visible"() -> (w532:bool)
        n316 = And(x=w533, y=w532) -> (x .and. y?=w528:bool)
        n317 = Select(t=u8 0 ("Disabled"), s=w533, f=u8 2) -> (s? t:f=w536:u8)
        n318 = Select(t=u8 0 ("Disabled"), s=w528, f=u8 2) -> (s? t:f=w529:u8)
        n319 = Bundle By Name(cluster=w538, "Cursor.Cursor Visible"=w533) -> (w537:T2)
        n320 = property on="Cursor Info.Visible" class="Bool (strict)"("Disabled"=w536) -> ()  [unwired: 2 in, 2 out]
        n321 = property on="Cursor Info Position.Lock" class="Bool (strict)"("Disabled"=w529) -> ()  [unwired: 2 in, 2 out]
      }
      event "Cursor.Color": Value Change {
        w539 = T17[] [enum."[Cursor] Apearance"] items=["None", "[Axis] Autoscale", "[Image] Update", "[Cursor] Name", "[Plot] Grid&BG", "[Marker] Update", "[Tree] Tags", "[Data] Update", "[Layout] Size", "[Tree] Checkbox", "[Tree] Visible", "[Tree] Open", "[Axis] X", "[Axis] Y", "[Plot] Color", "[Axis] Format String", "[Data] Compare Strings", "[Cursor] Apearance", "[Axis] Name&Visible", "[Tree] Color", "[Data] Index", "[Cursor] Index", "[Axis] Event"]
        n322 = event-data() -> ("NewVal"=w540:u32)  [unwired: 1 in]
        n323 = Bundle By Name(cluster=w542, "Cursor.Cursor Color"=w540) -> (w541:T2)
      }
      event "Marker.Point Style": Value Change {
        w543 = T17[] [enum."[Marker] Update"] items=["None", "[Axis] Autoscale", "[Image] Update", "[Cursor] Name", "[Plot] Grid&BG", "[Marker] Update", "[Tree] Tags", "[Data] Update", "[Layout] Size", "[Tree] Checkbox", "[Tree] Visible", "[Tree] Open", "[Axis] X", "[Axis] Y", "[Plot] Color", "[Axis] Format String", "[Data] Compare Strings", "[Cursor] Apearance", "[Axis] Name&Visible", "[Tree] Color", "[Data] Index", "[Cursor] Index", "[Axis] Event"]
        w554 = bool[] []
        n324 = event-data() -> ("CtlRef"=w545:refnum<vi>, "OldVal"=w546:T9, "NewVal"=w547:T9)  [unwired: 1 in]
        n325 = Variant To Data(type=w554, Variant=w547) -> (data=w553:bool[])  [unwired: 1 in, 1 out]
        n326 = Variant To Data(type=w554, Variant=w546) -> (data=w552:bool[])  [unwired: 1 in, 1 out]
        n327 = Exclusive Or(1:w553, 2:w552) -> (0:w551:bool[])
        n328 = Search 1D Array(1D array=w551, element=TRUE) -> (index of element=w544:i32)  [unwired: 1 in]
        n329 = Bundle By Name(cluster=w549, "Marker Point Style"=w544) -> (w548:T2)
        n330 = call <vilib>:"svx_SC Line Manage Cluster.vi"("index"=w544, "Clust Refnum"=w545) -> ()  [unwired: 10 in]
      }
      event "Marker Color": Value Change {
        w555 = T17[] [enum."[Marker] Update"] items=["None", "[Axis] Autoscale", "[Image] Update", "[Cursor] Name", "[Plot] Grid&BG", "[Marker] Update", "[Tree] Tags", "[Data] Update", "[Layout] Size", "[Tree] Checkbox", "[Tree] Visible", "[Tree] Open", "[Axis] X", "[Axis] Y", "[Plot] Color", "[Axis] Format String", "[Data] Compare Strings", "[Cursor] Apearance", "[Axis] Name&Visible", "[Tree] Color", "[Data] Index", "[Cursor] Index", "[Axis] Event"]
        n331 = event-data() -> ("NewVal"=w556:u32)  [unwired: 1 in]
        n332 = Bundle By Name(cluster=w558, "Marker Color"=w556) -> (w557:T2)
      }
      event "Marker.Visible": Value Change {
        w559 = T17[] [enum."[Marker] Update"] items=["None", "[Axis] Autoscale", "[Image] Update", "[Cursor] Name", "[Plot] Grid&BG", "[Marker] Update", "[Tree] Tags", "[Data] Update", "[Layout] Size", "[Tree] Checkbox", "[Tree] Visible", "[Tree] Open", "[Axis] X", "[Axis] Y", "[Plot] Color", "[Axis] Format String", "[Data] Compare Strings", "[Cursor] Apearance", "[Axis] Name&Visible", "[Tree] Color", "[Data] Index", "[Cursor] Index", "[Axis] Event"]
        n333 = event-data() -> ("NewVal"=w560:bool)  [unwired: 1 in]
        n334 = Bundle By Name(cluster=w562, "Maker Visible"=w560) -> (w561:T2)
      }
      event "Start Point": Value Change {
        n335 = event-data() -> ("NewVal"=w571:u16)  [unwired: 1 in]
        n336 = local read "Pair Selection"() -> (w565:u16)
        n337 = Unbundle By Name(w573) -> ("clearance boundary"=w575:T13, "pair index"=w567:i32[])
        n338 = Index Array(array=w567) -> (element=w566:i32)  [unwired: 1 in]
        n339 = Not Equal?(x=w565, y=w566) -> (x != y?=w564:bool)
        n340 = local read "Scale Fit"() -> (w563:bool)
        n341 = case shown="False" w564 {
          tunnel: [w577 _] -> w568
          tunnel: w563 -> [w576 _]
          frame False {
            w577 = T17[] [enum."[Axis] Autoscale", enum."[Image] Update"] items=["None", "[Axis] Autoscale", "[Image] Update", "[Cursor] Name", "[Plot] Grid&BG", "[Marker] Update", "[Tree] Tags", "[Data] Update", "[Layout] Size", "[Tree] Checkbox", "[Tree] Visible", "[Tree] Open", "[Axis] X", "[Axis] Y", "[Plot] Color", "[Axis] Format String", "[Data] Compare Strings", "[Cursor] Apearance", "[Axis] Name&Visible", "[Tree] Color", "[Data] Index", "[Cursor] Index", "[Axis] Event"]
            n342 = property on="Update Scale?" class="Bool (strict)"("Val(Sgnl)"=w576) -> ()  [unwired: 2 in, 2 out]
          }
          frame True {
          }
        }
        n343 = Index Array(array=w575, index=w565) -> (element=w570:T14)
        n344 = Bundle By Name(cluster=w570, "start point"=w571) -> (w569:T14)
        n345 = Replace Array Subset(array=w575, new element=w569, index=w565) -> (w574:T13)
        n346 = Bundle By Name(cluster=w573, "clearance boundary"=w574) -> (w572:T2)
      }
      event "X Axis": Value Change {
        n347 = event-data() -> ("NewVal"=w585:dbl)  [unwired: 1 in]
        n348 = local read "Pair Selection"() -> (w580:u16)
        n349 = Unbundle By Name(w588) -> ("clearance boundary"=w590:T13, "pair index"=w581:i32[])
        n350 = Index Array(array=w581) -> (element=w582:i32)  [unwired: 1 in]
        n351 = Not Equal?(x=w580, y=w582) -> (x != y?=w579:bool)
        n352 = local read "Scale Fit"() -> (w578:bool)
        n353 = Index Array(array=w590, index=w580) -> (element=w586:T14)
        n354 = Bundle By Name(cluster=w586, "boundary.x axis"=w585) -> (w584:T14)
        n355 = case shown="False" w579 {
          tunnel: [w592 _] -> w583
          tunnel: w578 -> [w591 _]
          frame False {
            w592 = T17[] [enum."[Axis] Autoscale", enum."[Image] Update"] items=["None", "[Axis] Autoscale", "[Image] Update", "[Cursor] Name", "[Plot] Grid&BG", "[Marker] Update", "[Tree] Tags", "[Data] Update", "[Layout] Size", "[Tree] Checkbox", "[Tree] Visible", "[Tree] Open", "[Axis] X", "[Axis] Y", "[Plot] Color", "[Axis] Format String", "[Data] Compare Strings", "[Cursor] Apearance", "[Axis] Name&Visible", "[Tree] Color", "[Data] Index", "[Cursor] Index", "[Axis] Event"]
            n356 = property on="Update Scale?" class="Bool (strict)"("Val(Sgnl)"=w591) -> ()  [unwired: 2 in, 2 out]
          }
          frame True {
          }
        }
        n357 = Replace Array Subset(array=w590, new element=w584, index=w580) -> (w589:T13)
        n358 = Bundle By Name(cluster=w588, "clearance boundary"=w589) -> (w587:T2)
      }
      event "Y Axis": Value Change {
        n359 = event-data() -> ("NewVal"=w600:dbl)  [unwired: 1 in]
        n360 = local read "Pair Selection"() -> (w595:u16)
        n361 = Unbundle By Name(w603) -> ("clearance boundary"=w605:T13, "pair index"=w596:i32[])
        n362 = Index Array(array=w596) -> (element=w597:i32)  [unwired: 1 in]
        n363 = Not Equal?(x=w595, y=w597) -> (x != y?=w594:bool)
        n364 = local read "Scale Fit"() -> (w593:bool)
        n365 = Index Array(array=w605, index=w595) -> (element=w601:T14)
        n366 = Bundle By Name(cluster=w601, "boundary.y axis"=w600) -> (w599:T14)
        n367 = case shown="False" w594 {
          tunnel: [w607 _] -> w598
          tunnel: w593 -> [w606 _]
          frame False {
            w607 = T17[] [enum."[Axis] Autoscale", enum."[Image] Update"] items=["None", "[Axis] Autoscale", "[Image] Update", "[Cursor] Name", "[Plot] Grid&BG", "[Marker] Update", "[Tree] Tags", "[Data] Update", "[Layout] Size", "[Tree] Checkbox", "[Tree] Visible", "[Tree] Open", "[Axis] X", "[Axis] Y", "[Plot] Color", "[Axis] Format String", "[Data] Compare Strings", "[Cursor] Apearance", "[Axis] Name&Visible", "[Tree] Color", "[Data] Index", "[Cursor] Index", "[Axis] Event"]
            n368 = property on="Update Scale?" class="Bool (strict)"("Val(Sgnl)"=w606) -> ()  [unwired: 2 in, 2 out]
          }
          frame True {
          }
        }
        n369 = Replace Array Subset(array=w605, new element=w599, index=w595) -> (w604:T13)
        n370 = Bundle By Name(cluster=w603, "clearance boundary"=w604) -> (w602:T2)
      }
      event "Pair Selection": Value Change {
        n371 = event-data() -> ("NewVal"=w610:u16)  [unwired: 1 in]
        n372 = Unbundle By Name(w608) -> ("clearance boundary"=w609:T13)
        n373 = Index Array(array=w609, index=w610) -> (element=w611:T14)
        n374 = Unbundle By Name(w611) -> ("start point"=w612:enum16{"center", "top", "bottom"}, "boundary.x axis"=w614:dbl, "boundary.y axis"=w613:dbl)
        n375 = local write "Start Point"(w612) -> ()
        n376 = local write "X Axis"(w614) -> ()
        n377 = local write "Y Axis"(w613) -> ()
      }
      event "Description": Value Change {
        n378 = event-data() -> ("NewVal"=w616:string)  [unwired: 1 in]
        n379 = property class="Ctl"(reference=w617, "Desc"=w616) -> ()  [unwired: 1 in, 2 out]
      }
      event "Tip strip": Value Change {
        n380 = event-data() -> ("NewVal"=w619:string)  [unwired: 1 in]
        n381 = property class="Ctl"(reference=w620, "TipStrip"=w619) -> ()  [unwired: 1 in, 2 out]
      }
      event "Update Scale?": Value Change {
        n382 = event-data() -> ()  [unwired: 1 in, 1 out]
        n383 = local read "Scale Selection"() -> (w624:u16)
        n384 = case shown="1" w624 {
          tunnel: w621 -> [w628 w631]
          tunnel: [w627 w630] -> w623
          tunnel: [w626 w629] -> w622
          frame 0, Default {
            n385 = Unbundle By Name(w628) -> ("X Scale.Maximum"=w627:dbl, "X Scale.Minimum"=w626:dbl)
          }
          frame 1 {
            n386 = Unbundle By Name(w631) -> ("Y Scale.Maximum"=w630:dbl, "Y Scale.Minimum"=w629:dbl)
          }
        }
        n387 = local write "Update Scale?"(FALSE ("Update Scale?")) -> ()
        n388 = local write "Minimum"(w622) -> ()
        n389 = local write "Maximum"(w623) -> ()
      }
    }
    n390 = call <vilib>:"svx_SC Line Event Consumer.vi"("shaft centerline"=w148, "State in"=w151, "events"=w149, "references"=w145) -> ("State out"=w150:T2)  [unwired: 7 in]
  }
  "Action out" <- w12
  "State Out" <- w10
